vi "SNK3_HF.vi"() -> ()   [LabVIEW 2017]
uses:
  Control_EU/AScan5.ctl
  Control_EU/AScanXY.ctl
  <vilib>/Utility/error.llb/DialogType.ctl
  Control_EU/DataCluster.ctl
  Control_EU/UNDT_ClusterPackRevers (Type).ctl
  E:/_git/LV_Unicorn/Control/unicorn_Param.ctl
  E:/_git/LV_Unicorn/Control/unicorn_conn.ctl
  E:/_git/LV_Unicorn/Control/unicorn_JSON.ctl
  E:/_git/LV_Unicorn/Control/unicorn_ParamInt.ctl
  E:/_git/LV_Unicorn/Control/unicorn_Telemetry.ctl
  E:/_git/LV_Unicorn/Control/unicorn_Table.ctl
  E:/_git/LV_Unicorn/Control/unicorn_ParamFloat.ctl
  Control_EU/UNDT_Graph (Type).ctl
  Control_EU/MeasControl2.ctl
  Control_EU/FilterCor (Type).ctl
  <vilib>/Utility/miscctls.llb/LVPositionTypeDef.ctl
  <vilib>/Utility/miscctls.llb/LVBoundsTypeDef.ctl
  <vilib>/Utility/miscctls.llb/LVRowAndColumnTypeDef.ctl
  E:/_git/LV_Unicorn/LV_Unicorn.lvlib
panel:
  out "Table":string[][](table)
  out "Overload":bool[](array[boolean])
  in  "ScaleAbciss":enum16{"Время", "Растояние"}(ring) caption="Ось X"
  in  "AutoScaleTime":bool=TRUE caption="Автомасштаб оси X"
  out "AScanXY":T1 caption="XY Graph - Light"
  out "AScan 2":T2=[{"f0"=0.0, "df"=1.999999987845058e-08, "magnitude"=[-8.362428618581513, -16.48524282862701, -13.270215291464396, -1.44247262127071, -0.14146356256599724, -51.99620101896437, -99.78053816073843, -95.12827294380126, -90.88869610452232, -90.57171306559249, -87.25341160556846, -85.8105891846696, -82.76337415652955, -80.86227527247217, -78.40234828439452, -76.19434956898783, -74.01576834598359, -71.78529755390673, -69.68513234090051, -67.52084604331412, -65.28443000252219, -63.28035098812552, -61.47587187035788, -55.13083503627922, -33.66107495355482, -4.448097020118439, 6.700743833810975, -2.283159610513394, -7.84886632585858, 20.366429733203404, 85.31206280454444, 128.55518730024505, 126.6691916223117, 121.44842700443678, 120.34183392161685, 117.1312140668606, 115.09733972218146, 112.07993143953263, 109.58979749310856, 106.99556091118939, 104.39191050125919, 101.93090119993394, 99.39922086918887, 96.97715585938386, 94.53860842694485, 92.13340433368103, 89.79334219186057, 87.4974982431977, 84.36064872487259, 79.96205068879135, 75.24407280826563, 69.6830936007591, 63.012279743985346, 56.68454128407484, 50.848901457596185, 45.15521557730699, 39.80757945206551, 34.87529947330404, 30.326640668357868, 25.873379055661644, 21.437604126664155, 17.226033165145054, 13.29233985936753, 9.51676315482473, 5.868301535314458, 2.6152379190580177, -0.17432084983738605, -2.9230732928817815, -5.72915589706281, -8.184331474023566, -10.351473082454504, -12.583499883397053, -14.78807691482325, -16.80357569484977, -18.681385196647625, -20.315395063160395, -21.635529485686448, -23.060485075707675, -24.67995225859704, -25.990605155052435, -26.962380226163987, -27.8979823545651, -28.73810296071838, -29.462829936045352, -30.316506058786985, -31.231589134722654, -31.90290135924215, -32.28940013073094, -32.56549527286779, -32.84419147253834, -33.10821799085829, -33.304481879338255, -33.46348407210644, -33.725072745996385, -33.968450151919114, -34.08677302658134, -34.095260888540906, -33.808795901495614, -33.460191943170685, -33.34710648415603, -33.31294418132484, -33.164550879301714, -32.76087185762208, -32.24668349645117, -31.870751672834558, -31.59434042822022, -31.322524907283878, -30.987392928483132, -30.54575777807395, -29.960390802933034, -29.194569385082104, -28.35521615897005, -27.62954955178202, -27.16065053686043, -26.837023014710212, -26.337914212675514, -25.71672342288184, -25.366631450281602, -25.0282208409094, -24.10622696739074, -22.93802219334293, -22.196530061297835, -21.860867523784236, -21.48748057143621, -20.868178290548485, -20.258140316942672, -19.741215960041927, -19.043028419689563, -18.327886007838515, -17.88242873042077, -17.410982641516057, -16.751452435353258, -16.108829161595168, -15.466698716435872, -14.79714242030252, -14.15875938689237, -13.51766704991087, -13.037019622874197, -12.883695422881942, -12.688494826915928, -12.003125979495529, -11.041384732025477, -10.084146598250413, -9.094988080956, -8.456447500145373, -8.350068617135094, -8.081518682681917, -7.434963428810079, -6.886095277938921, -6.459481766096815, -6.006742309917172, -5.620911678318862, -5.31553427736344, -4.833348073185789, -4.023214092920625, -3.34493790122724, -3.164730433913519, -2.9873376703399117, -2.3525611732443394, -1.6414614161376448, -1.1393857023135752, -0.7026244223184221, -0.32843603777837416, 0.05392266421858949, 0.5455805395231437, 1.1545903160676971, 1.781017592099488, 2.1783846355274363, 2.3977169397439866, 2.665823543012266, 2.9966959607709214, 3.26432535821732, 3.308674526046161, 3.253305179315248, 3.4221076308822376, 3.869108561619214, 4.335963537628231, 4.5814517046546825, 4.784279759130186, 5.183043868629284, 5.453526093130677, 5.427387813380847, 5.645768572191628, 6.244742510133619, 6.7991138215475075, 7.095702891390829, 7.047903714554195, 7.022261210930083, 7.424905424799363, 7.751004705825835, 7.762319244342507, 7.964564695372246, 8.341866396149271, 8.5654588424768, 8.684667654972145, 8.910024715720283, 9.320113816427693, 9.681328111244511, 9.82042605812967, 9.932776687086516, 10.142521316622151, 10.358957614276733, 10.506859328193968, 10.57077349352403, 10.546141368829922, 10.328487343140296, 10.07575920412637, 10.415274780592881, 11.094160586595535, 11.1505633923789, 10.86742877213328, 10.912559327658528, 11.057356953535418, 11.039702429150566, 10.996767826725772, 11.0376960190315, 11.103126869322296, 11.209970057860119, 11.313258819693147, 11.284415966702, 11.287074491221574, 11.317094694615662, 11.153033313477863, 11.164239905021532, 11.507872766702349, 11.54247437227059, 11.245325654941553, 11.284050122036206, 11.60608735389178, 11.684968277664666, 11.552378091289938, 11.30140977616611, 10.82661768874459, 10.552244657690608, 10.730994969471794, 10.877123869724528, 10.799195529112694, 10.689736112373794, 10.550420705492797, 10.323919095222664, 10.143144721401768, 10.238665189584935, 10.300660044676988, 9.877206661005403, 9.430313941227723, 9.375324885704686, 9.274215891535277, 8.97357832792477, 8.962562153335966, 9.31708468024408, 9.395592837025106, 8.951893496609046, 8.490135195852417, 8.349086505424566, 8.490678117530479, 8.621734183776425, 8.474382694063024, 8.254557446893159, 8.08427593174929, 8.008460564436973, 8.166791542098508, 8.139075587574553, 7.846901022328893, 7.817067734629745, 7.839851256288966, 7.585179076138957, 7.335045937828909, 7.162006690912676, 6.940819550198285, 6.836077513955388, 6.936004569442957, 7.062421923523289, 7.029144812631785, 6.8410717702354304, 6.693133085989757, 6.576838506898639, 6.415406266518403, 6.460329048099084, 6.8260616523512, 7.063685025475934, 6.830997901977753, 6.540760553090877, 6.413424153006417, 5.958987769712621, 5.3708356607021415, 5.388070204628093, 5.699517827597447, 5.705195043963613, 5.641944201379374, 5.799467017764982, 5.970988142689748, 5.807005608165127, 5.3246424658118485, 4.860039317596602, 4.624090649915161, 4.646748362163635, 4.749191009974311, 4.680270924636716, 4.500713930749043, 4.367592408763812, 4.225989613421916, 4.151125465745281, 4.213723680311887, 4.159140027255489, 4.002432062387015, 3.952611752314624, 3.957092286027546, 3.8829357749400515, 3.6539695825686067, 3.4836802273675858, 3.423265760191498, 3.2487988787561335, 3.1556659578109247, 3.1891273339861073, 3.007045679469229, 2.6904212670106062, 2.479388271780408, 2.341186118315818, 2.287069402584166, 2.304384948052757, 2.119308207078575, 1.6629850131757848, 1.4292599067393894, 1.5348852188617457, 1.4873002503245516, 1.3294569906902325, 1.3013776101597614, 1.2726427204106585, 1.1502594846460852, 0.7491829966038495, 0.24296145992775564, 0.21561241826202604, 0.41891116519582283, 0.27361930057122663, 0.05490456389088649, 0.06342031008716731, 0.023829591709727538, -0.12211693620702135, -0.10022365821896528, 0.13808831118331, 0.2572844946789701, -0.038020760019207955, -0.451183307570318, -0.46499836947805306, -0.17207548691658303, -0.11017842560977442, -0.3275198146511684, -0.46812528558439226, -0.4643833141108189, -0.35511715348184225, -0.2316420424176613, -0.24180173921013193, -0.28982339790672995, -0.40532542428081797, -0.5930137058367109, -0.66422549393792, -0.7359407593976357, -0.7426463673255057, -0.5872296669112984, -0.5528867670263935, -0.6206878161829081, -0.6536080379892155, -0.5933601194583389, -0.4043312653657267, -0.34505391499988036, -0.4973056554072173, -0.6806381473443253, -0.8142567518480064, -0.7602558335283902, -0.6034238278398334, -0.6499078635251863, -0.8511098952358225, -1.0372637329319332, -1.0373002243404699, -0.8003105749385213, -0.7355750021488348, -0.9524111472992445, -1.150236596544346, -1.209007262785235, -1.1337058391754908, -1.1860405047445965, -1.4007784850109601, -1.536762599852409, -1.6860273416677956, -1.6924470009635115, -1.4112204348384694, -1.3699058167276235, -1.7008180109278328, -1.9213176048579044, -2.110995081726287, -2.3202647740099565, -2.0249377193167675, -1.5526853836036025, -1.5086623250890625, -1.6033312274894342, -1.8652128730554978, -2.4902599231427303, -2.9286209145266184, -2.8737155718090435, -2.6342273377531455, -2.4779406172337985, -2.535840186173118, -2.6692602695266032, -2.589781662843052, -2.4953836821823643, -2.700424055835356, -2.9828725086108534, -3.0823670179938745, -3.0936821349923775, -3.045846607479234, -2.89969529082191, -2.8673928842927126, -2.8816708087679217, -2.654989520570325, -2.4880829681678733, -2.6582434162510253, -2.8447974560167495, -2.835933851381469, -2.792141705112954, -2.844217979802579, -2.906390653235121, -2.86229991317623, -2.7575688328979595, -2.604821473637003, -2.4683593096679033, -2.5354120137767495, -2.6219441167590958, -2.52585252828203, -2.3582229980534066, -2.0089848048764907, -1.589152812267912, -1.6895458889016481, -2.3193483221029965, -2.7390600744138283, -2.5632325668843805, -2.3299278921913356, -2.3886126672950923, -2.3424710799840796, -2.3113094003665537, -2.544097375845922, -2.6177735194071374, -2.4038119720510167, -2.104478329481708, -1.8769032436987345, -1.8297884165408504, -1.8397176026994657, -1.9241985213398038, -2.172246434820863, -2.3580485310660606, -2.350211338635063, -2.2969404170673897, -2.266134637073719, -2.1596259798795927, -2.0569351767576336, -2.1042590716192535, -2.1498693061028007, -2.259218623822335, -2.5957630417007067, -2.8766772717946196, -2.7582052913397774, -2.249975786520963, -1.9910433550871858, -2.2452515904476513, -2.4381017241790914, -2.4313391339662758, -2.226923331641842, -1.9012009420130198, -2.024960099043483, -2.4015471209291945, -2.4217247349968716, -2.398582307210802, -2.5954482817147664, -2.637866804554733, -2.4530357145601442, -2.264939520810856, -2.2922411154767133, -2.6196098565765737, -2.901625679773872, -2.878426945936468, -2.608991094906088, -2.2387857641482753, -2.09453085314685, -2.204732517612733, -2.2719190011368156, -2.3166224061620517, -2.286914558026254, -2.1429486168223733, -2.3244217551271618, -2.688567341423635, -2.5972807503556226, -2.216139264306605, -1.9378262417934877, -1.7862010187935766, -1.8305964693306578, -1.9965156460901028, -2.086063208620317, -1.9612220244869718, -1.6455034137032385, -1.5811718615387917, -1.781927054860887, -1.7300633286956213, -1.5254276131966549, -1.4552768078465874, -1.4523745520051534, -1.4914536016906368, -1.5893559168812885, -1.6015688051501797, -1.3944289829226477, -1.2666103232660362, -1.388013237006021, -1.4446035143943163, -1.4962791866852285, -1.6908152736442617, -1.7476937379832407, -1.5876830010743106, -1.2777607982993686, -1.017954355658162, -1.1298205385137408, -1.2730121585939287, -1.0632148179361138, -0.8644639282300659, -1.0099510796040931, -1.3206230134837824, -1.5056142446026115, -1.4862541127040458, -1.3769159774615218, -1.2309918205446593, -1.0234725791449364, -0.9411732883463628, -0.9697684889927132, -0.9517257621215549, -1.0898865632028674, -1.3386563353294605, -1.4914969798998072, -1.5830446476098814, -1.5645732343650707, -1.4580894296914266, -1.3227021722798327, -1.2047299034683192, -1.3215155550166173, -1.482586656757917, -1.359866040902034, -1.1772395757790264, -0.9929342830718042, -0.8774222730518204, -1.1099924327160124, -1.3080030773072622, -1.2084609742055363, -1.2499391622181975, -1.5056830886296666, -1.4185389284449457, -0.9615123969335855, -0.7803563936448654, -0.9576656839298039, -1.2740004999209305, -1.5303181849230896, -1.4469397956454486, -1.2210108533554376, -1.0927434475643167, -1.0887609884819085, -1.1768500340380115, -1.1383812615431452, -0.899624876448911, -0.7467888409761372, -0.8332742820899739, -0.9191905856778249, -0.8735255850086787, -0.620948668965184, -0.20360162817735272, -0.004829021887644558, -0.06126518615371879, -0.1206794575970207, -0.13042972371681572, -0.14361233031024767, -0.23623177455158384, -0.3409376971964093, -0.37580386508943775, -0.3756449052634707, -0.30167336121257904, -0.15735143907022575, -0.18575377039746854, -0.5125215808075154, -0.6710384180156552, -0.40567774298176573, -0.2658003113576797, -0.3670234725342425, -0.3873427200990136, -0.5013808185888138, -0.6775818427701097, -0.7093324148102056, -0.6240102187909997, -0.31594965771523675, -0.056491991648499607, -0.3432900902159872, -0.7960975868587639, -0.6535675952762858, -0.22854146809868325, -0.29192425843518777, -0.5485119771361724, -0.538319443776345, -0.567697080604944, -0.648059770870077, -0.4951732810517342, -0.2539965079262174, -0.1450610284459799, -0.3003100969881416, -0.7128360258332123, -1.079760020695403, -1.0787566074927781, -0.6326880874656808, -0.10784068463988206, 0.0343957311192753, -0.06698642450328407, -0.13309667361363609, -0.3163761163689287, -0.5315324135831361, -0.3813514187557985, -0.054354728121325024, -0.01385841181718206, -0.16997792231552467, -0.3121017327842992, -0.3990411551312718, -0.36364339922238287, -0.3396735727582154, -0.3071585842604918, -0.010359696911223182, 0.14511950447445088, -0.2589224126552381, -0.5762151230680956, -0.43965938793621717, -0.24733515444995646, -0.19387261615293028, -0.3351491608715378, -0.34532398299666056, -0.027889339253533763, 0.12939961103563746, 0.056654333865026274, 0.1230607529222425, 0.18840971818906382, 0.023524623384787446, 0.007162268968954777, 0.23430478795387444, 0.2837222544059159, 0.17897281281159394, 0.031042575950152695, -0.32807431300739154, -0.7136821519388832, -0.6748008976255733, -0.3134642003245176, -0.005201762167928337, 0.28332615312939424, 0.4825814929413923, 0.4382697634825945, 0.3363950751918878, 0.33043354091955734, 0.4245915317824256, 0.49330159180635746, 0.4035130214653009, 0.24375024460977102, 0.11354505150364957, 0.02126287245380354, -0.053544948000080694, -0.13859926601122652, -0.0724822990500229, 0.20118154548850953, 0.2683717810496091, -0.02587055520410786, -0.3496768753386732, -0.41745076228284006, -0.16421334153824318, 0.12033453428193752, 0.25209620468524463, 0.28430791817811496, 0.18264540514900318, 0.049018916363763765, 0.0016300540045790513, 0.0181018425878392, -0.012450352299282486, -0.26050342961477213, -0.6106594874185305, -0.5902151022163196, -0.16157144082393415, 0.1913050218443857, 0.3467194083880827, 0.3594821624047597, 0.25514771482377796, 0.14863756867879374, 0.02526945654861379, -0.030411099402272157, -0.057532872068520646, -0.1678352196447861, 0.0050842552622896164, 0.4679356219693602, 0.4775913842308057, 0.03565776707866064, -0.02192071464214962, 0.3637345593877086, 0.5089700224787066, 0.21595635766497878, -0.08851796028834258, -0.11535308413340317, 0.07008582549362075, 0.3172098958150116, 0.42725851306396123, 0.19434939967916165, -0.17960096836732475, -0.22300681125435062, 0.03684553140349678, 0.23990696494710662, 0.23882353609518603, 0.2197403890365326, 0.3719346251314626, 0.5769936938241691, 0.5824062303123618, 0.3189435134705114, 0.12519266613720959, 0.16463577053156797, 0.19030497718591022, 0.13549962363308055, 0.13201797751310806, 0.23932364475072632, 0.35005152851859833, 0.3373705359796446, 0.20432943219903166, 0.052721705922394335, 0.10298776022501954, 0.3701207427268116, 0.5430249736029396, 0.5009148342087713, 0.2978760718557538, 0.09219321070600017, 0.13393330859835828, 0.33953567960239184, 0.43052035242115494, 0.38148098994517454, 0.415351558669272, 0.4582932174478742, 0.3124023389633237, 0.17299399106730107, -0.07635904591123222, -0.5307978843140688, -0.5929384987070989, -0.20434243019323617, 0.030884435369358698, -0.011348368912109663, 0.0029669081454244406, 0.14538493119147233, 0.21417009991179725, 0.31184163814498334, 0.371777860209761, 0.1056468743233836, -0.14466540253590665, -0.18406641780580912, -0.32792074087453216, -0.26237246641650813, 0.2894105244412515, 0.6608584286579742, 0.5052543644725347, 0.1611669455267588, -0.12816430138968826, -0.19007337823893522, 0.07215810742349049, 0.5163022496016083, 0.7510023125434486, 0.5472167454923351, 0.32134272812413656, 0.31761231132520606, 0.18537161733263474, 0.03675229199535579, 0.2337274456237992, 0.4585991394025086, 0.3415603897793176, 0.09129735788513926, 0.0756513488759083, 0.21255672357818867, 0.09540049811892004, -3.0665706674426474e-05, 0.2852105377101566, 0.3755848838875977, 0.2018957983494829, 0.1774616682042165, 0.06773902100451323, 0.04379244419664019, 0.3463110501602955, 0.3871378118556663, 0.1833799034141066, 0.2670117046574205, 0.3980808418215247, 0.4290106422002964, 0.458031160928158, 0.27521104721830625, 0.12677865244972963, 0.35520975234021535, 0.5952039721412348, 0.42272504463551286, 0.16031661647281226, 0.21580758179447912, 0.2812243238033716, 0.21902584997582153, 0.3035538101453312, 0.3863830045150394, 0.2917921304942297, 0.28192564587595825, 0.3600489951124928, 0.29434435160408157, 0.1764079844710409, 0.15126766455074403, 0.1763195440069012, 0.04668268981527035, -0.3192578279350755, -0.46618615472317515, -0.14601272298170898, 0.11839185082453696, 0.046519034135144466, -0.042003371722159955, 0.1733477203089251, 0.34455614839816917, -0.07812140797659595, -0.4820299265186918, -0.365581182070855, -0.3375999362822881, -0.5159617905794676, -0.4801205776030315, -0.0732860204226995, 0.4390020279794271, 0.5500131027357611, 0.3648195836488526, 0.20158268236087906, 0.052373137554127425, 0.04563646472297478, 0.05242342103815645, -0.05843066410290021, 0.12945128198407474, 0.5201484582841545, 0.526558984370638, 0.2815502865862527, 0.1492985192964511, 0.10739855659323894, 0.09861915156182022, -0.04135048827669152, -0.35717774361660304, -0.49062788692197046, -0.3209427930853508, 0.016743293250272018, 0.45027484979311794, 0.6216169483678868, 0.4066347156396546, 0.27828313162228824, 0.4707579866840206, 0.6751239786804035, 0.5663001391731655, 0.2615591431004418, 0.14383809871912945, 0.27329166712002007, 0.3410492437734547, 0.3084481169778428, 0.4179537195461194, 0.6732638998383322, 0.8377463664749598, 0.6077008571803617, 0.12627074749883604, -0.030575282680729288, 0.019599161533733422, -0.10365977653168557, -0.12553792707120692, -0.0769794053737769, -0.1637377197200749, -0.09915977471496262, 0.045841608370267295, 0.14535723523528077, 0.3531225340724973, 0.2927312182763444, -0.08970625436268165, -0.15144323159029227, 0.038091603654322626, 0.18762153296160022, 0.3619296478664751, 0.2715231920734027, 0.07013930077545183, 0.20351536174541707, 0.2577293424268987, -0.02410580504505333, -0.2208582024454131, -0.24358480952264472, -0.29277281265297006, -0.316985698973383, -0.20252234111882217, -0.029825552761167273, 0.07774714092482782, 0.11932168624412043, 0.11986880273639144, 0.024756918557329755, -0.20753617553964432, -0.31491271309062085, -0.12032840126028077, 0.01836648590835921, -0.017545829771620447, 0.04954906309080798, 0.1353245450206373, 0.015480990582943832, -0.14787166808844177, -0.057943116083833957, 0.23473363006445425, 0.4173171072892501, 0.512254784727304, 0.6156594232339785, 0.4157091926279577, -0.059021886098150844, -0.2608760366894103, -0.1091841671644147, -0.053648216270971716, -0.11989447865158809, -0.04507068097427691, -0.06597328023218552, -0.2045302059898404, 0.06697666428232196, 0.4984994216806058, 0.384164441988446, 0.016536383149343692, -0.04917977024359743, 0.08319316914810315, 0.08657038669196027, -0.13275948959216066, -0.2077937299213204, 0.007552074793011343, 0.10345140142192122, 0.01329369268262326, 0.08062963424987402, 0.2863543156377659, 0.20276990257247007, -0.13826596361974453, -0.2547753602261764, -0.08288696976654819, 0.08417466470160662, 0.06835279501615332, 0.044575476585407614, 0.033416567190897695, -0.1368734589356677, -0.21416558183864254, -0.1492720501744884, -0.06898489334548685, -0.07289999506372169, -0.26528800995998836, -0.21049792023552527, 0.013814347194966103, -0.09401329989805163, -0.262602759939341, -0.2616421759547052, -0.10424188169645277, 0.10439958779164726, 0.175354545824689, 0.2173334881438791, 0.19286862516662495, 0.1412484277265662, 0.12012481576584833, -0.15301161441982458, -0.4815057561094136, -0.45341131556318715, -0.1445173348590174, 0.1663094149535027, 0.2099185189720174, -0.07742022745577515, -0.41168006577396454, -0.45924723795656064, -0.2756570382527457, -0.17081435490473496, -0.1693257181831882, -0.0786346890587879, 0.15919665769553148, 0.3773983729545307, 0.3759213188999979, 0.09973732479323871, -0.17066898838561428, 0.027740917095059103, 0.34729937252632226, 0.18999857876508486, -0.10778459345812053, -0.23149832753205146, -0.17943298052233558, 0.10809672363149048, 0.37739306215007673, 0.5303181336562943, 0.5814618677817407, 0.3888715199087187, 0.10232232585565271, -0.13786434062996022, -0.24750633688256585, -0.1203930974364198, -0.04723627025555288, -0.1252965541626736, -0.046062891273265905, 0.15716680469029143, 0.216832061463208, -0.08796584481672198, -0.4652283810208928, -0.2605998533882712, 0.10981870056053822, -0.003628019655366188, -0.08618401606685211, 0.09732282934305658]}, ...(72 in all)]
  in  "FreqFind":dbl=-1.0 caption="Частота, МГц" min=-1.0 max=10000000.0 format="%_3f"
  out "UNDT_meas":string[][](table)=[["Частота, Гц", "1", "-", "-"], ["СКЗ, В", "1", "-", "-"], ["Амплитуда, В", "1", "-", "-"], ["Амплитуда, дБмкВ", "1", "-", "-"], ["Датчик пути 1, мм", "1", "-", "-"], ["Датчик пути 2, мм", "1", "-", "-"], ["Время, сек", "1", "-", "-"]]
  in  "Tab":enum32{"Параметры общие", "Отладка", "K"}(tab)=enum."K"
  in  "Автозапрос телеметри":bool
  in  "Тип детектора":enum16{"Оконный детектор", "Гильберт"}(ring)=enum."Гильберт"
  in  "FiltrCor":bool caption="Поправка на АЧХ фильтра"
  in  "speed":dbl=1500.0 caption="скорость звука, м/с"
  in  "DelaiProtector":dbl[](array[numeric])=[0.0, 0.0, 0.0, 0.0, 0.0, 0.0, 0.0, 0.0, 0.0, 0.0, 0.0, 0.0, 0.0, 0.0, 0.0, 0.0, 0.0, 0.0, 0.0, 0.0, 0.0, 0.0, 0.0, 0.0, 0.0, 0.0, 0.0, 0.0, 0.0, 0.0, 0.0, 0.0, 0.0, 0.0, 0.0, 0.0, 0.0, 0.0, 0.0, 0.0, 0.0, 0.0, 0.0, 0.0, 0.0, 0.0, 0.0, 0.0, 0.0, 0.0, 0.0, 0.0, 0.0, 0.0, 0.0, 0.0, 0.0, 0.0, 0.0, 0.0, 0.0, 0.0, 0.0, 0.0] caption="Задержка в проетекторе, мкс"
  out "HPF_Bode":cluster{"Frq":dbl[], "Kt":dbl[]}[](graph)=[{"Frq"=[100000.0, 200000.0, 300000.0, 400000.0, 500000.0, 600000.0, 700000.0, 800000.0, 900000.0, 1000000.0, 1100000.0, 1200000.0, 1300000.0, 1400000.0, 1500000.0, 2000000.0, 3000000.0, 4000000.0, 5000000.0, 6000000.0, 7000000.0, 8000000.0, 9000000.0, 10000000.0, 11000000.0, 12000000.0, 13000000.0, 14000000.0, 15000000.0], "Kt"=[0.37286, 0.79297, 0.90962, 0.95419, 0.97594, 0.98749, 0.98845, 0.99808, 1.00096, 1.00096, 1.00192, 1.00192, 1.00289, 1.00289, 1.00192, 1.0, 0.98653, 0.96728, 0.94447, 0.91646, 0.8898, 0.85438, 0.80953, 0.76035, 0.69865, 0.62859, 0.54832, 0.46631, 0.38142]}, {"Frq"=[100000.0, 200000.0, 300000.0, 400000.0, 500000.0, 600000.0, 700000.0, 800000.0, 900000.0, 1000000.0, 1100000.0, 1200000.0, 1300000.0, 1400000.0, 1500000.0, 2000000.0, 3000000.0, 4000000.0, 5000000.0, 6000000.0, 7000000.0, 8000000.0, 9000000.0, 10000000.0, 11000000.0, 12000000.0, 13000000.0, 14000000.0, 15000000.0], "Kt"=[0.3742, 0.79565, 0.91266, 0.95739, 0.97874, 0.99034, 0.9971, 1.00097, 1.00386, 1.0029, 1.00483, 1.00483, 1.00483, 1.00483, 1.00386, 1.0, 0.98068, 0.94986, 0.90947, 0.85923, 0.79836, 0.72744, 0.6486, 0.56483, 0.47855, 0.39459, 0.31478, 0.24271, 0.18]}, {"Frq"=[100000.0, 200000.0, 300000.0, 400000.0, 500000.0, 600000.0, 700000.0, 800000.0, 900000.0, 1000000.0, 1100000.0, 1200000.0, 1300000.0, 1400000.0, 1500000.0, 2000000.0, 3000000.0, 4000000.0, 5000000.0, 6000000.0, 7000000.0, 8000000.0, 9000000.0, 10000000.0, 11000000.0, 12000000.0, 13000000.0, 14000000.0, 15000000.0], "Kt"=[0.37978, 0.80756, 0.9262, 0.97125, 0.99215, 1.00393, 1.01079, 1.01374, 1.01178, 1.01472, 1.01472, 1.01472, 1.01374, 1.01178, 1.01079, 1.0, 0.96222, 0.90903, 0.84171, 0.76408, 0.67763, 0.58508, 0.49117, 0.3999, 0.31452, 0.23886, 0.17399, 0.12139, 0.08052]}, {"Frq"=[100000.0, 200000.0, 300000.0, 400000.0, 500000.0, 600000.0, 700000.0, 800000.0, 900000.0, 1000000.0, 1100000.0, 1200000.0, 1300000.0, 1400000.0, 1500000.0, 2000000.0, 3000000.0, 4000000.0, 5000000.0, 6000000.0, 7000000.0, 8000000.0, 9000000.0, 10000000.0, 11000000.0, 12000000.0, 13000000.0, 14000000.0, 15000000.0], "Kt"=[1.0, 1.0, 1.0, 1.0, 1.0, 1.0, 1.0, 1.0, 1.0, 1.0, 1.0, 1.0, 1.0, 1.0, 1.0, 1.0, 1.0, 1.0, 1.0, 1.0, 1.0, 1.0, 1.0, 1.0, 1.0, 1.0, 1.0, 1.0, 1.0]}, {"Frq"=[], "Kt"=[]}]
  in  "Захват потока":bool
  out "IndCntr":u32
  in  "BasePathData":path=path "D:/YandexDisk/!Work/_labview/SNK3/data"
  in  "ZeroDimensionDetect":i32=10
  out "MD5_filter_ini":string="528970cebd473443910cf3af22e246ff"
  in  "UNDT_HF_Filter":u16=7 caption="ФВЧ аппаратный" max=10 step=1
  in  "I_AMP1_PE2":i32
  in  "I_AMP1_PE1":i32
  out "ScaleADC":bool=TRUE
  in  "StartLen":T3={"start samples/time"=0.0, "duration"=7e-05, "EnableSubset"=FALSE}
  out "LPF_Bode":cluster{"Frq":dbl[], "Kt":dbl[]}[](graph)=[{"Frq"=[100000.0, 200000.0, 300000.0, 400000.0, 500000.0, 600000.0, 700000.0, 800000.0, 900000.0, 1000000.0, 1100000.0, 1200000.0, 1300000.0, 1400000.0, 1500000.0, 2000000.0, 3000000.0, 4000000.0, 5000000.0, 6000000.0, 7000000.0, 8000000.0, 9000000.0, 10000000.0, 11000000.0, 12000000.0, 13000000.0, 14000000.0, 15000000.0], "Kt"=[0.37335, 0.7928, 0.90924, 0.95331, 0.97471, 0.98638, 0.99416, 0.99805, 1.00097, 1.0, 1.00195, 1.00195, 1.00195, 1.00195, 1.00195, 1.0, 0.98735, 0.96848, 0.94484, 0.91946, 0.89125, 0.86021, 0.82772, 0.79426, 0.75934, 0.72539, 0.69066, 0.65661, 0.62296]}, {"Frq"=[100000.0, 200000.0, 300000.0, 400000.0, 500000.0, 600000.0, 700000.0, 800000.0, 900000.0, 1000000.0, 1100000.0, 1200000.0, 1300000.0, 1400000.0, 1500000.0, 2000000.0, 3000000.0, 4000000.0, 5000000.0, 6000000.0, 7000000.0, 8000000.0, 9000000.0, 10000000.0, 11000000.0, 12000000.0, 13000000.0, 14000000.0, 15000000.0], "Kt"=[0.37335, 0.7928, 0.90924, 0.95331, 0.97471, 0.98638, 0.99416, 0.99805, 1.00097, 1.0, 1.00195, 1.00195, 1.00195, 1.00195, 1.00195, 1.0, 0.98735, 0.96848, 0.94484, 0.91946, 0.89125, 0.86021, 0.82772, 0.79426, 0.75934, 0.72539, 0.69066, 0.65661, 0.62296]}, {"Frq"=[100000.0, 200000.0, 300000.0, 400000.0, 500000.0, 600000.0, 700000.0, 800000.0, 900000.0, 1000000.0, 1100000.0, 1200000.0, 1300000.0, 1400000.0, 1500000.0, 2000000.0, 3000000.0, 4000000.0, 5000000.0, 6000000.0, 7000000.0, 8000000.0, 9000000.0, 10000000.0, 11000000.0, 12000000.0, 13000000.0, 14000000.0, 15000000.0], "Kt"=[0.37335, 0.7928, 0.90924, 0.95331, 0.97471, 0.98638, 0.99416, 0.99805, 1.00097, 1.0, 1.00195, 1.00195, 1.00195, 1.00195, 1.00195, 1.0, 0.98735, 0.96848, 0.94484, 0.91946, 0.89125, 0.86021, 0.82772, 0.79426, 0.75934, 0.72539, 0.69066, 0.65661, 0.62296]}, {"Frq"=[100000.0, 200000.0, 300000.0, 400000.0, 500000.0, 600000.0, 700000.0, 800000.0, 900000.0, 1000000.0, 1100000.0, 1200000.0, 1300000.0, 1400000.0, 1500000.0, 2000000.0, 3000000.0, 4000000.0, 5000000.0, 6000000.0, 7000000.0, 8000000.0, 9000000.0, 10000000.0, 11000000.0, 12000000.0, 13000000.0, 14000000.0, 15000000.0], "Kt"=[0.37335, 0.7928, 0.90924, 0.95331, 0.97471, 0.98638, 0.99416, 0.99805, 1.00097, 1.0, 1.00195, 1.00195, 1.00195, 1.00195, 1.00195, 1.0, 0.98735, 0.96848, 0.94484, 0.91946, 0.89125, 0.86021, 0.82772, 0.79426, 0.75934, 0.72539, 0.69066, 0.65661, 0.62296]}, {"Frq"=[100000.0, 200000.0, 300000.0, 400000.0, 500000.0, 600000.0, 700000.0, 800000.0, 900000.0, 1000000.0, 1100000.0, 1200000.0, 1300000.0, 1400000.0, 1500000.0, 2000000.0, 3000000.0, 4000000.0, 5000000.0, 6000000.0, 7000000.0, 8000000.0, 9000000.0, 10000000.0, 11000000.0, 12000000.0, 13000000.0, 14000000.0, 15000000.0], "Kt"=[0.20101, 0.60917, 0.79214, 0.87772, 0.9244, 0.95111, 0.96794, 0.97883, 0.98639, 0.98962, 0.99325, 0.99567, 0.99728, 0.99849, 0.99919, 1.0, 0.98871, 0.97006, 0.94536, 0.91804, 0.8877, 0.85474, 0.82046, 0.78558, 0.7497, 0.71522, 0.68054, 0.64677, 0.61381]}, {"Frq"=[100000.0, 200000.0, 300000.0, 400000.0, 500000.0, 600000.0, 700000.0, 800000.0, 900000.0, 1000000.0, 1100000.0, 1200000.0, 1300000.0, 1400000.0, 1500000.0, 2000000.0, 3000000.0, 4000000.0, 5000000.0, 6000000.0, 7000000.0, 8000000.0, 9000000.0, 10000000.0, 11000000.0, 12000000.0, 13000000.0, 14000000.0, 15000000.0], "Kt"=[0.20101, 0.60917, 0.79214, 0.87772, 0.9244, 0.95111, 0.96794, 0.97883, 0.98639, 0.98962, 0.99325, 0.99567, 0.99728, 0.99849, 0.99919, 1.0, 0.98871, 0.97006, 0.94536, 0.91804, 0.8877, 0.85474, 0.82046, 0.78558, 0.7497, 0.71522, 0.68054, 0.64677, 0.61381]}, {"Frq"=[100000.0, 200000.0, 300000.0, 400000.0, 500000.0, 600000.0, 700000.0, 800000.0, 900000.0, 1000000.0, 1100000.0, 1200000.0, 1300000.0, 1400000.0, 1500000.0, 2000000.0, 3000000.0, 4000000.0, 5000000.0, 6000000.0, 7000000.0, 8000000.0, 9000000.0, 10000000.0, 11000000.0, 12000000.0, 13000000.0, 14000000.0, 15000000.0], "Kt"=[0.20101, 0.60917, 0.79214, 0.87772, 0.9244, 0.95111, 0.96794, 0.97883, 0.98639, 0.98962, 0.99325, 0.99567, 0.99728, 0.99849, 0.99919, 1.0, 0.98871, 0.97006, 0.94536, 0.91804, 0.8877, 0.85474, 0.82046, 0.78558, 0.7497, 0.71522, 0.68054, 0.64677, 0.61381]}, {"Frq"=[100000.0, 200000.0, 300000.0, 400000.0, 500000.0, 600000.0, 700000.0, 800000.0, 900000.0, 1000000.0, 1100000.0, 1200000.0, 1300000.0, 1400000.0, 1500000.0, 2000000.0, 3000000.0, 4000000.0, 5000000.0, 6000000.0, 7000000.0, 8000000.0, 9000000.0, 10000000.0, 11000000.0, 12000000.0, 13000000.0, 14000000.0, 15000000.0], "Kt"=[0.20101, 0.60917, 0.79214, 0.87772, 0.9244, 0.95111, 0.96794, 0.97883, 0.98639, 0.98962, 0.99325, 0.99567, 0.99728, 0.99849, 0.99919, 1.0, 0.98871, 0.97006, 0.94536, 0.91804, 0.8877, 0.85474, 0.82046, 0.78558, 0.7497, 0.71522, 0.68054, 0.64677, 0.61381]}]
  in  "ScaleOrdinate":T4(ring)=enum."Вольты" caption="Ось ординат"
  out "Log":string="[8:41:50] Запуск ПО СНК3. Версия 2.0.30032026. Цифровой идентификатор (MD5):  .\r\n"
  in  "SaveParam":bool
  in  "GainCompens":bool
  out "Ошибка":bool
  in  "UDPDataInd0":bool
  in  "save_osc":bool[](array[boolean])
  in  "index_osc":i32=32
  in  "Refresh":bool
  in  "RingMenu":u16(ring) items=["Основные параметры", "Данные", "Параметры фильтра", "Прочее"]
  in  "TabRight":enum32{"Page 1", "Page 4", "Page 3", "Page 2"}(tab)
  in  "TxPulseCh0":u8=1 caption="№ ПЭП подкл. к ГИВ" min=1 max=16 step=1
  in  "TxPulseCh1":u8=1 caption="Кол-во имп. ГИ" min=1 max=16 step=1
  in  "HPF_Filter_Prog":T5(ring)=enum."Выкл." caption="ФВЧ"
  in  "TxDelay1":dbl caption="t задержки имп., мкс" min=0.0 max=30.0 step=0.05 format="%.2g"
  in  "TxCh0":u8=1 caption="№ ПЭП подкл. к ГИВ" min=1 max=8 step=1
  in  "WPulse0":dbl=0.4000000059604645 caption="t импульса, мкс" min=0.05 max=1.0 step=0.01 format="%.2g"
  in  "Tx0":bool=TRUE caption="Разрешить работу генератора"
  in  "TxDelay0":dbl caption="t задержки имп. , мкс" min=0.0 max=30.0 step=0.05 format="%.2g"
  in  "Tick":i32=1 caption="№ такта" min=1 max=32 step=1
  in  "TxCh1":u8=16 caption="№ ПЭП подкл. к ГИ" min=9 max=16 step=1
  in  "Tx1":bool=TRUE caption="Разрешить работу генератора"
  in  "PWhite1":dbl=0.4000000059604645 caption="t импульса, мкс" min=0.05 max=1.0 step=0.01 format="%_2g"
  in  "RxCh0":u8=1 caption="№ ПЭП подкл. к приемнику" min=1 max=8 step=1
  in  "RxDelay0":dbl caption="t задержки разв. , мкс" min=0.0 max=200.0 step=1.0
  in  "RxCh1":u8=9 caption="№ ПЭП подкл. к приемнику" min=9 max=16 step=1
  in  "RxDelay1":dbl caption="t задержки разв. , мкс" min=0.0 max=200.0 step=1.0
  in  "Rx0":bool=TRUE caption="Разрешить работу приемника"
  in  "Rx1":bool=TRUE caption="Разрешить работу приемника"
  in  "RxWhite0":dbl=20.0 caption="t разв. , мкс" min=1.0 max=80.0
  in  "RxWhite1":dbl=20.0 caption="t разв. , мкс" min=1.0 max=80.0
  in  "Gain1":dbl caption="Усиление, дБ" min=0.0 max=80.0 step=1.0
  in  "Gain0":dbl caption="Усиление, дБ" min=0.0 max=80.0 step=1.0
  in  "UNDT_Mean":i32=4 caption="Усреднение по времени" min=0 max=28 step=4
  in  "UNDT_NTick":i32=1 caption="Количество тактов" min=1 max=32 step=1
  in  "UNDT_Freq":i32=100 caption="Частота следования тактов, Гц" min=20 max=1000 step=1
  in  "UNDT_GIV2":T6(ring)=enum."60" caption="Амплитуда ГИВ2 (ПЭП 9...16), В"
  in  "UNDT_GIV1":T6(ring)=enum."60" caption="Амплитуда ГИВ1 (ПЭП 1...8), В"
  in  "Type_signal":T7(ring)
  in  "LPF_Filter":enum16{"14 МГц", "10 МГц", "7.5 МГц"}(ring) caption="ФНЧ"
  in  "Видеофильтр":bool=TRUE
  in  "TrigLevel":dbl=0.1 caption="Уровень триггера" min=-1.0 max=10000000.0 format="%_3f"
  in  "IIR filter":T8={"Topology"=enum."Butterworth", "Type"=enum."Bandpass", "Order"=4, "Lower Fc"=300000.0, "Upper Fc"=15000000.0, "PB Ripple"=3.0, "SB Attenuation"=60.0} {"PB Ripple" format="%0.2f"; "SB Attenuation" format="%0.2f"; "Lower Fc" format="%0.2p"; "Upper Fc" format="%0.2p"}
  in  "IndEnqu":enum16{"NoEnqu", "LossyEnqu", "Enqu"}(ring)=enum."LossyEnqu"
  in  "Interpolation factor (n)":i32=1
  in  "Ind":bool=TRUE
  in  "max queue size":i32=4
  out "UpTime":sgl
  in  "Connect":bool
  in  "Save":bool
  in  "Pause":bool
  in  "UNDT_Start":bool
  # "График 1"
  # "График 2"
  # "График 3"
  # "График 4"
  # "График 5"
  # "График 6"
  # "График 7"
  # "График 8"
  # "ПЭП 1...8"
  # "ПЭП 9...16"
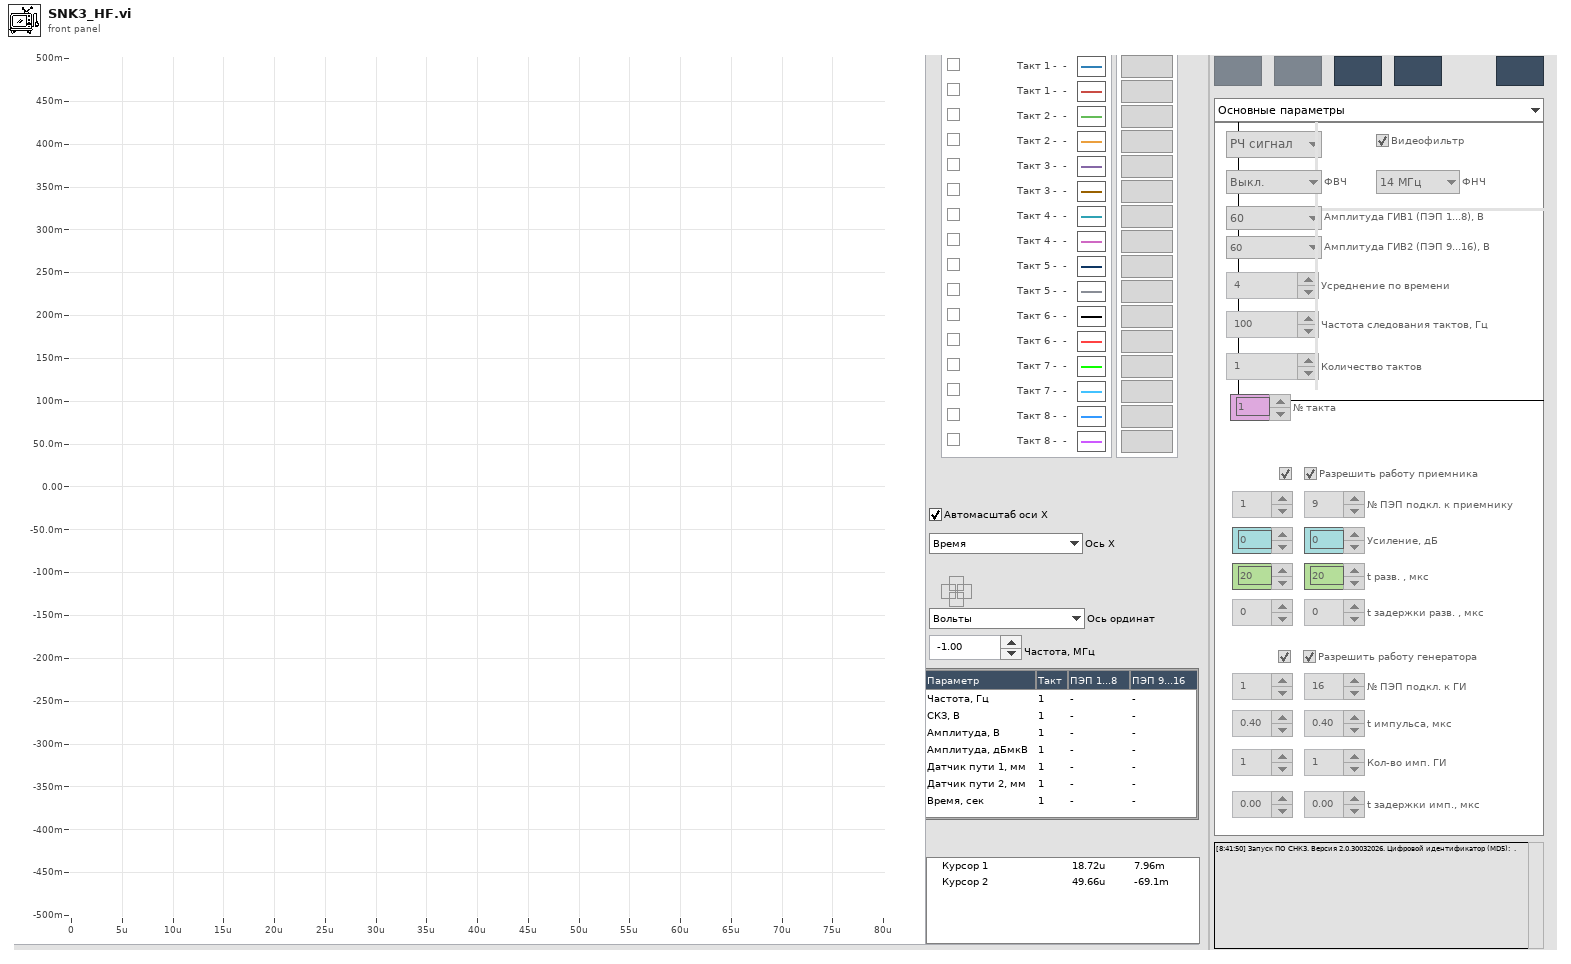
[diagram p1: front panel]
types:
  T1 = typedef "AScanXY.ctl" = cluster{dbl[], dbl[]}[]
  T2 = typedef "AScan5.ctl" = cluster{"f0":dbl, "df":dbl, "magnitude":dbl[]}[]
  T3 = cluster{"start samples/time":dbl, "duration":dbl, "EnableSubset":bool}
  T4 = enum16{"Отсчеты АЦП (±32767)", "Проценты", "Вольты", "дБмкВ (отн. 1 мкВ)", "Отсчеты АЦП (±1)"}
  T5 = enum16{"0.4 МГц", "0.8 МГц", "1.5 МГц", "2.0 МГц", "Выкл."}
  T6 = enum16{"20", "40", "60", "80", "100", "120", "140", "160", "180", "200"}
  T7 = enum16{"РЧ сигнал", "Детект. полное", "Положит.", "Отрицат."}
  T8 = cluster{"Topology":enum16{"Off", "Butterworth", "Chebyshev", "Inverse Chebyshev", "Elliptic", "Bessel"}, "Type":enum16{"Lowpass", "Highpass", "Bandpass", "Bandstop"}, "Order":i32, "Lower Fc":dbl, "Upper Fc":dbl, "PB Ripple":dbl, "SB Attenuation":dbl}
  T9 = typedef "LV_Unicorn.lvlib/unicorn_Param.ctl" = cluster{"conParam":T10, "Param":T11}
  T10 = typedef "LV_Unicorn.lvlib/unicorn_conn.ctl" = cluster{"ReadIntParam":bool, "ReadDescrParam":bool, "ReadFloatParam":bool, "debug":bool, "ReadJSON":bool, "IP_address":string, "N_attempts":i32, "type_con":enum16{"Serial", "TCP"}, "MB_address":i32, "VISA":refnum<visa-resource-name>, "connection ID":refnum<k5>, "nameDevices":string, "timeout":i32, "port":u16, "type_version":string, "baud_rate":u32, "VersionControl":bool, "TCP_conn":bool, "WindowSize":i32}
  T11 = typedef "LV_Unicorn.lvlib/unicorn_JSON.ctl" = cluster{"NumParam":cluster{"NTelem":i32, "NInt":i32, "NFloat":i32, "NTable":i32}, "ParamInt":T12, "Telemetry":T13, "Table":T14, "ParamFloat":T15}
  T12 = typedef "LV_Unicorn.lvlib/unicorn_ParamInt.ctl" = cluster{"ID":string, "Num":i32, "Name":string, "Type":string, "Enum":string, "Desc":string, "Unit":string, "Access":string, "FormatStr":string, "Min":i32, "Max":i32}[]
  T13 = typedef "LV_Unicorn.lvlib/unicorn_Telemetry.ctl" = cluster{"ID":string, "Num":i32, "Name":string, "Desc":string, "Unit":string, "FormatStr":string, "Min":i32, "Max":i32}[]
  T14 = typedef "LV_Unicorn.lvlib/unicorn_Table.ctl" = cluster{"Num":i32, "Access":string, "ColumnCount":i32, "NeedParamPrepare":bool, "Columns":cluster{"Column":i32, "Desc":string, "Name":string}[], "DataType":string, "FormatStr":string, "ID":string, "Name":string, "RowCount":i32, "Rows":cluster{"Desc":string, "ID":string, "Max":i32, "Min":i32, "Name":string, "Row":i32, "Unit":string}[], "Type":string}[]
  T15 = typedef "LV_Unicorn.lvlib/unicorn_ParamFloat.ctl" = cluster{"ID":string, "Num":i32, "Name":string, "Type":string, "Enum":string, "Desc":string, "Unit":string, "Access":string, "FormatStr":string, "Min":sgl, "Max":sgl}[]
  T16 = typedef "DataCluster.ctl" = cluster{"UNDT_Cluster":T17, "UNDT_Cluster_Data":dbl[]}
  T17 = typedef "UNDT_ClusterPackRevers (Type).ctl" = cluster{"PacketCounter":u32, "Gain Coeff":sgl, "SamplingInterval":sgl, "Lose Packet":u32, "EncodersParam2":u64, "EncodersParam1":u64, "Reserve 1":u8, "Mux TX/RX":u8, "ScanDelay":u16, "CRC 8":u8, "ScanDuration":u16, "N chanel":u8, "GlobalTime2":u32, "GlobalTime1":u32, "N tick":u8, "Ncycle":u16, "FrameFormatVersion":u8, "MagicWord":u32, "Overload":bool}
  T18 = typedef "DialogType.ctl" = u16
  T19 = enum8{"Enabled", "Disabled", "Disabled and Grayed Out"}
  T20 = typedef "LVRowAndColumnTypeDef.ctl" = cluster{"Row":i32, "Column":i32}
  T21 = cluster{"Версия:":string, "Наименование ПО:":string, "Год выпуска:":string, "Производитель:":string, "MD5":string, "Наименование ПО полное:":string, "Build":string}
  T22 = typedef "ConfigINI.ctl" = cluster{"IP_PC":string, "IP_SNK3":string, "UDP_port_0":u32, "UDP_port_1":u32, "Serial_Code":string, "ADCToVoltage0":dbl, "DelayChN":dbl[], "GainCorrection":dbl[][], "CorCh":dbl[], "PulseCor":dbl[][], "ADCToVoltage1":dbl}
  T23 = typedef "OptionPACK5.ctl" = cluster{"MagicWordStr":string, "Header size":u32, "Проверка CRC8":bool, "Проверка конца пакета":bool, "GainCompens":bool, "Неотбрасывать BadEnd пакеты":bool, "Неотбрасывать BadCRC пакеты":bool, "Привести к 1":bool, "GainCoef":bool, "K_scale":dbl, "ScaleOrdinate":enum16{"Отсчеты АЦП (±32767)", "Проценты", "Вольты", "дБмкВ (отн. 1 мкВ)", "Отсчеты АЦП (±1)"}}
  T24 = enum16{"Отсчеты АЦП ", "Отсчеты АЦП приведенные к ±1", "Вольты", "дБмкВ (отн. 1 мкВ)"}
  T25 = typedef "LVPositionTypeDef.ctl" = cluster{"Left":i32, "Top":i32}
  T26 = typedef "LVBoundsTypeDef.ctl" = cluster{"Width":u32, "Height":u32}
  T27 = typedef "LVRangeTypeDef.ctl" = cluster{"Minimum":dbl, "Maximum":dbl, "Increment":dbl, "Minor Increment":dbl, "Start":dbl}
  T28 = typedef "LVRectTypeDef.ctl" = cluster{"Left":i16, "Top":i16, "Right":i16, "Bottom":i16}
  T29 = typedef "FilterCor (Type).ctl" = cluster{"HPFFilterNum":enum16{"HPF_OFF", "1", "2", "3", "4", "5", "6", "7", "8", "9", "10"}, "LPFBode":cluster{"Frq":dbl[], "Kt":dbl[]}[], "HPFBode":cluster{"Frq":dbl[], "Kt":dbl[]}[], "EnableFilterСorrect":bool, "LPF_Filter":enum16{"14 МГц", "10 МГц", "7.5 МГц", "Выкл."}}
  T30 = typedef "MeasControl2.ctl" = cluster{"approx freq":dbl, "search (+/- % of Fsampl.)":dbl, "start, duration":cluster{"start samples/time":dbl, "duration":dbl, "EnableSubset":bool}, "averaging type":enum16{"Linear", "Exponential"}, "window":enum16{"Rectangular (none)", "Hanning", "Low side lobe"}, "hysteresis":dbl, "level":dbl}
  T31 = typedef "UNDT_Graph (Type).ctl" = cluster{"UNDT_Type_signal":enum16{"РЧ сигнал", "Детект. полное", "Положит.", "Отрицат."}, "ФНЧ":bool, "UNDT_Mean":i32, "IIR filter":cluster{"Topology":enum16{"Off", "Butterworth", "Chebyshev", "Inverse Chebyshev", "Elliptic", "Bessel"}, "Type":enum16{"Lowpass", "Highpass", "Bandpass", "Bandstop"}, "Order":i32, "Lower Fc":dbl, "Upper Fc":dbl, "PB Ripple":dbl, "SB Attenuation":dbl}, "ZeroDimension":i32, "ТипДетектора":enum16{"Оконный детектор", "Гильберт"}, "FilterCor":cluster{"HPFFilterNum":enum16{"HPF_OFF", "1", "2", "3", "4", "5", "6", "7", "8", "9", "10"}, "LPFBode":cluster{"Frq":dbl[], "Kt":dbl[]}[], "HPFBode":cluster{"Frq":dbl[], "Kt":dbl[]}[], "EnableFilterСorrect":bool, "LPF_Filter":enum16{"14 МГц", "10 МГц", "7.5 МГц", "Выкл."}}, "MeasControl":T30}
  T32 = typedef "MeasControl.ctl" = cluster{"FFT amplitude":dbl, "amplitude":dbl, "RMS":dbl, "detected frequency":dbl, "way sensor 1":ext, "way sensor 2":ext, "detected frequency 2":dbl, "time trig":dbl, "time trig 2":dbl, "DC":dbl, "trigger detected?":bool, "FFT amplitude mean":dbl}
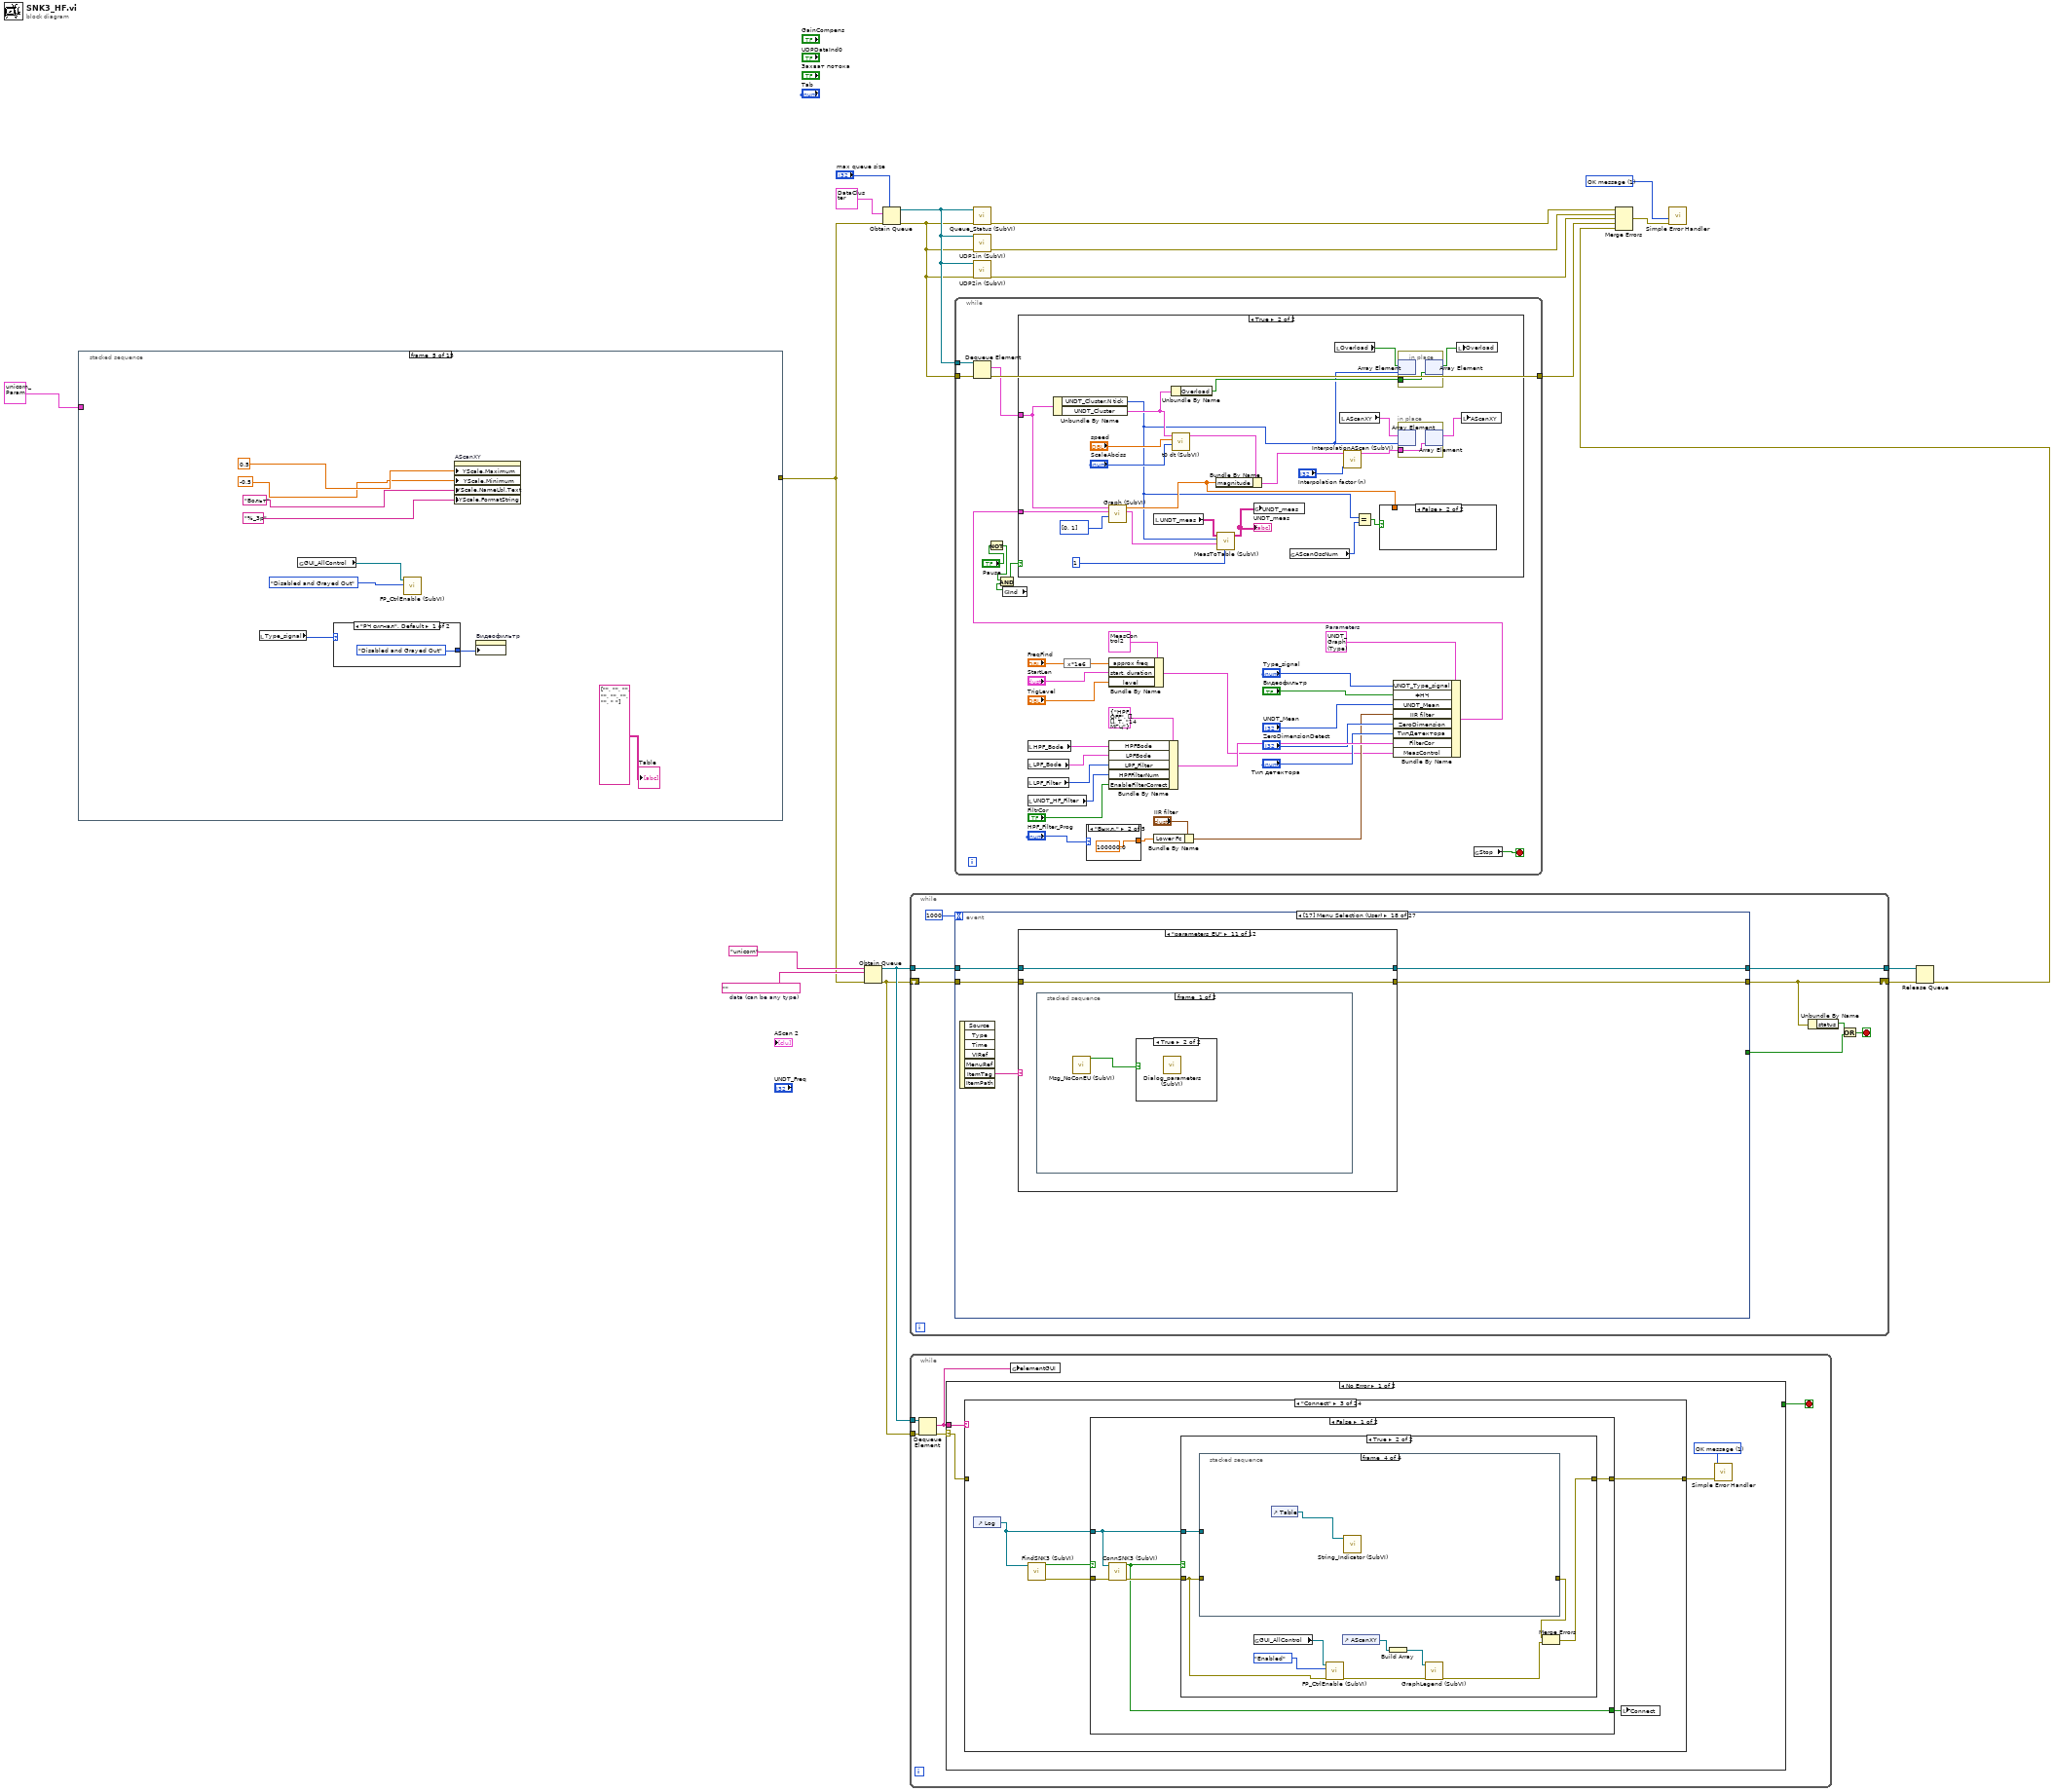
[diagram p0: block diagram]
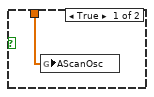
[diagram p3: hidden frame]
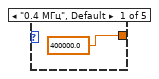
[diagram p4: hidden frame]
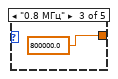
[diagram p5: hidden frame]
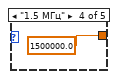
[diagram p6: hidden frame]
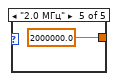
[diagram p7: hidden frame]
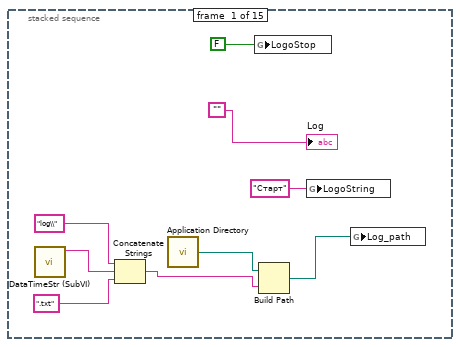
[diagram p8: hidden frame]
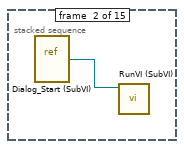
[diagram p9: hidden frame]
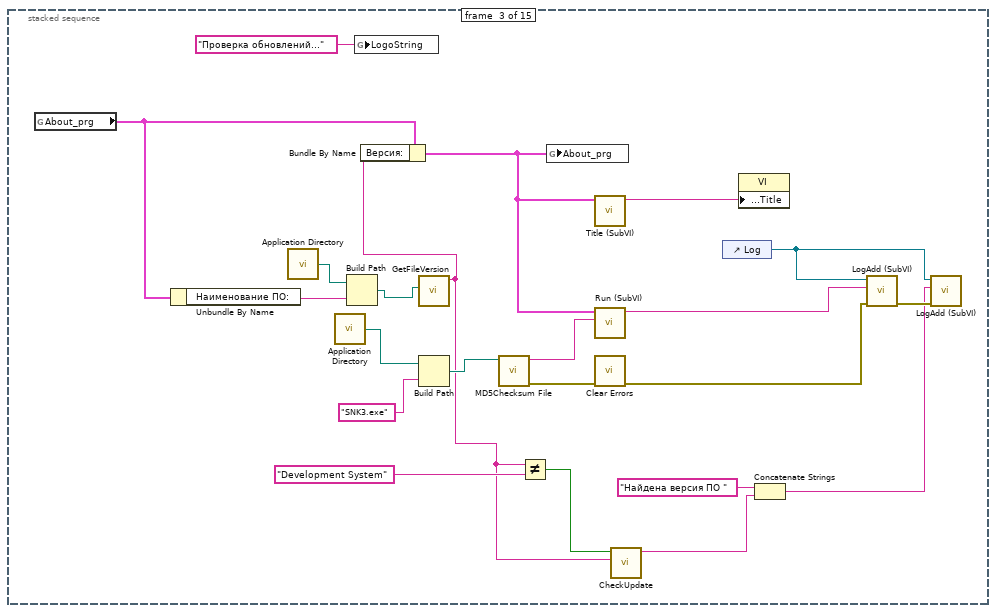
[diagram p10: hidden frame]
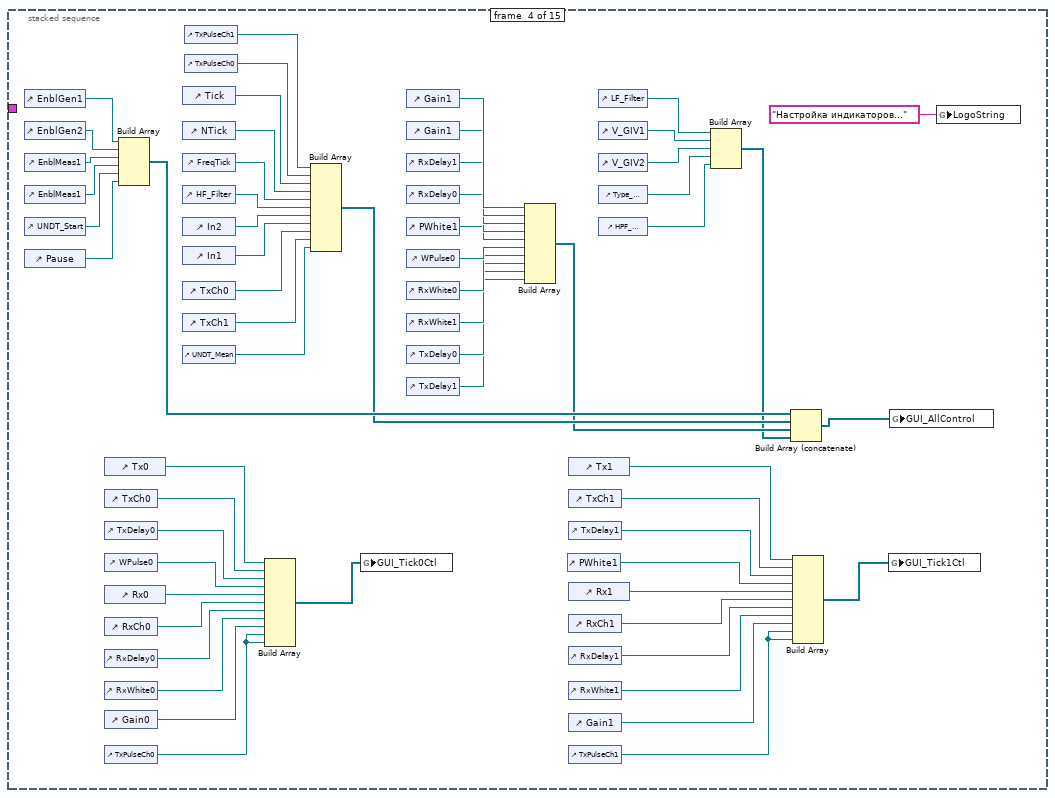
[diagram p11: hidden frame]
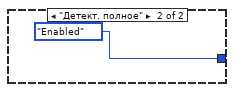
[diagram p12: hidden frame]
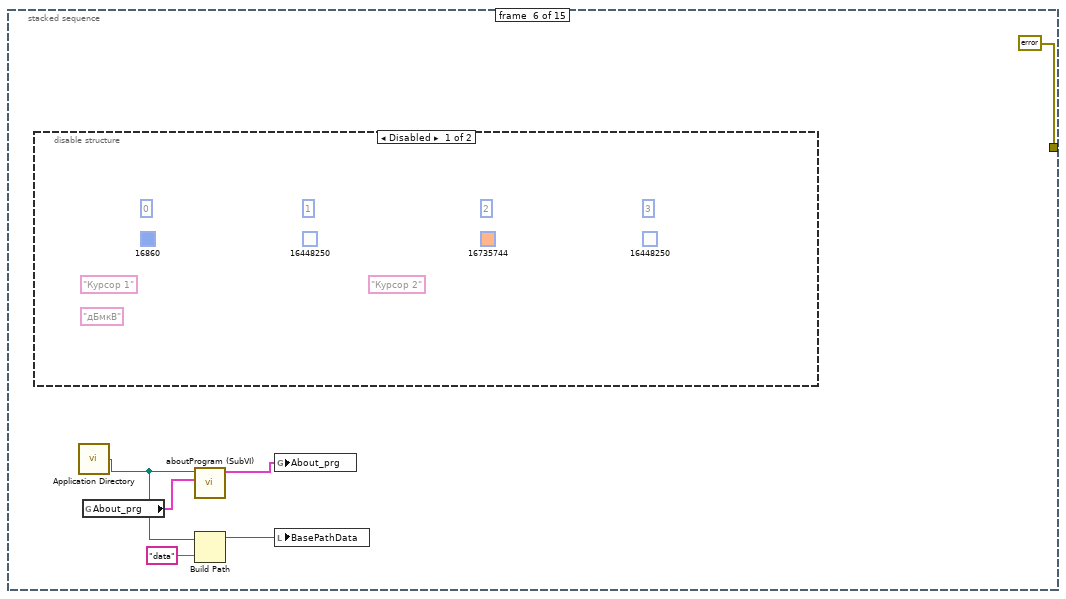
[diagram p13: hidden frame]
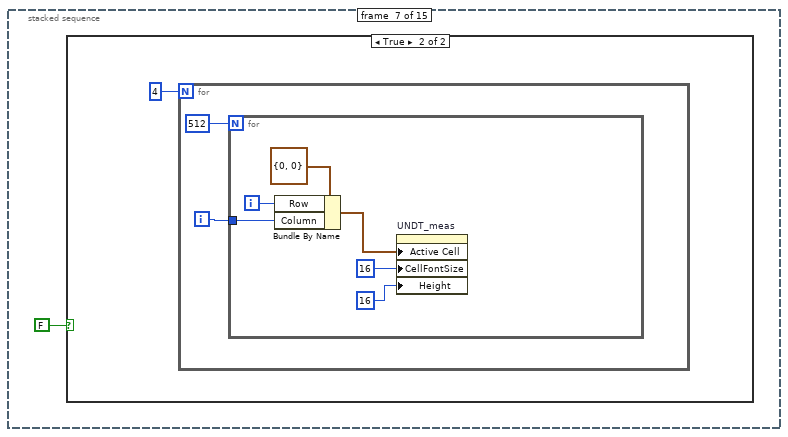
[diagram p15: hidden frame]
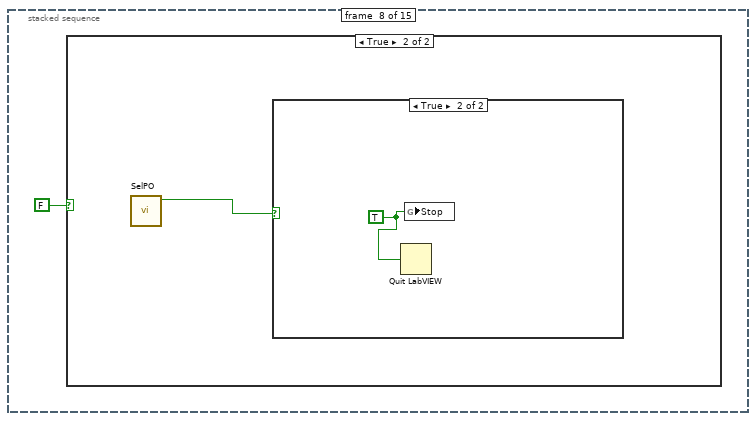
[diagram p17: hidden frame]
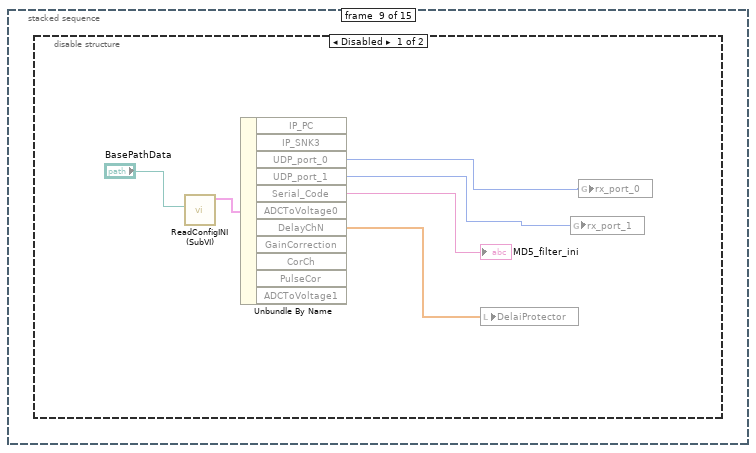
[diagram p20: hidden frame]
diagram:
  w18 = ""  # data (can be any type)
  w19 = T18 1 items=["no dialog", "OK message", "continue or stop message", "OK message + warnings", "continue/stop + warnings"] ("type of dialog (OK msg:1)")
  n1 = stacked-sequence {
    tunnel: [_ _ _ _ _ errorcluster {"status"=FALSE, "code"=0, "source"=""} ("error in (no error)") _ _ _ _ _ _ _ _ _] -> w3
    tunnel: T9 {"conParam"={"ReadIntParam"=TRUE, "ReadDescrParam"=FALSE, "ReadFloatParam"=TRUE, "debug"=FALSE, "ReadJSON"=TRUE, "IP_address"="192.168.1.216", "N_attempts"=5, "type_con"=enum."TCP", "MB_address"=1, "VISA"="COM1", "connection ID"=refnum, "nameDevices"="", "timeout"=2000, "port"=2000, "type_version"="0F0C0005", "baud_rate"=115200, "VersionControl"=TRUE, "TCP_conn"=FALSE, "WindowSize"=700}, "Param"={"NumParam"={"NTelem"=201, "NInt"=16, "NFloat"=10, "NTable"=2}, "ParamInt"=[], "Telemetry"=[], "Table"=[], "ParamFloat"=[]}} ("paramUnicorn") -> [_ _ _ _ _ _ _ _ _ _ w174 _ _ _ _]
    frame #0 {
      n2 = call "DataTimeStr (SubVI).vi"() -> ("DataTimeStr"=w23:string)  [unwired: 11 in]
      n3 = Concatenate Strings("log\\" ("name or relative path"), w23, ".txt" ("name or relative path")) -> (w22:string)
      n4 = call <vilib>:"Application Directory.vi"() -> ("Application Directory"=w24:path)
      n5 = global write "Global_SNK3_HF.vi" "LogoStop"(FALSE ("StopStartLogo")) -> ()
      n6 = Build Path(base path=w24, name or relative path=w22) -> (appended path=w25:path)
      n7 = global write "Global_SNK3_HF.vi" "LogoString"("Старт" ("LogoString")) -> ()
      n8 = global write "Global_SNK3_HF.vi" "Log_path"(w25) -> ()
      "Log" <- ""
    }
    frame #1 {
      n9 = vi-ref "Dialog_Start (SubVI).vi"() -> (w29:refnum<vi>)
      n10 = call "RunVI (SubVI).vi"("VI in"=w29) -> ()  [unwired: 11 in]
    }
    frame #2 {
      n11 = global read "Global_SNK3_HF.vi" "About_prg"() -> (w41:T21)
      n12 = Unbundle By Name(w41) -> ("Наименование ПО:"=w43:string)
      n13 = call <vilib>:"Application Directory.vi"() -> ("Application Directory"=w42:path)
      n14 = call <vilib>:"Application Directory.vi"() -> ("Application Directory"=w49:path)
      n15 = Build Path(base path=w42, name or relative path=w43) -> (appended path=w40:path)
      n16 = global write "Global_SNK3_HF.vi" "LogoString"("Проверка обновлений..." ("LogoString")) -> ()
      n17 = call "GetFileVersion.vi"("path"=w40) -> ("Full version"=w37:string)  [unwired: 10 in]
      n18 = Bundle By Name(cluster=w41, "Версия:"=w37) -> (w44:T21)
      n19 = Build Path(base path=w49, name or relative path="SNK3.exe") -> (appended path=w48:path)
      n20 = call <vilib>:"MD5Checksum File.vi"("Path"=w48) -> ("error out"=w45:errorcluster, "MD5 message-digest"=w47:string)  [unwired: 9 in]
      n21 = Not Equal?(x=w37, y="Development System" ("Full version")) -> (x != y?=w38:bool)
      n22 = global write "Global_SNK3_HF.vi" "About_prg"(w44) -> ()
      n23 = call "Title (SubVI).vi"("About_prg"=w44) -> ("String"=w46:string)  [unwired: 10 in]
      n24 = call "Run (SubVI).vi"("MD5 message-digest"=w47, "About_prg"=w44) -> ("String"=w51:string)  [unwired: 9 in]
      n25 = call <vilib>:"Clear Errors.vi"("error in (no error)"=w45) -> ("error out"=w30:errorcluster)  [unwired: 5 in, 1 out]
      n26 = call "CheckUpdate.vi"("Установленная версия ПО"=w37, "GitHub"=w38) -> ("Последняя версия ПО"=w32:string)  [unwired: 9 in]
      n27 = control-ref of="Log"() -> (w34:refnum<vi>)
      n28 = property class="VI"("Front Panel.Title"=w46) -> ()  [unwired: 2 in, 2 out]
      n29 = Concatenate Strings("Найдена версия ПО " ("string"), w32) -> (w31:string)
      n30 = call "LogAdd (SubVI).vi"("error in"=w30, "string"=w51, "Log"=w34) -> ("error out"=w35:errorcluster)  [unwired: 8 in]
      n31 = call "LogAdd (SubVI).vi"("error in"=w35, "string"=w31, "Log"=w34) -> ()  [unwired: 8 in, 1 out]
    }
    frame #3 {
      n32 = control-ref of="EnblGen1"() -> (w111:refnum<vi>)
      n33 = control-ref of="EnblGen2"() -> (w110:refnum<vi>)
      n34 = control-ref of="EnblMeas1"() -> (w109:refnum<vi>)
      n35 = control-ref of="EnblMeas1"() -> (w108:refnum<vi>)
      n36 = control-ref of="UNDT_Start"() -> (w78:refnum<vi>)
      n37 = control-ref of="Pause"() -> (w77:refnum<vi>)
      n38 = control-ref of="Tx0"() -> (w76:refnum<vi>)
      n39 = control-ref of="TxCh0"() -> (w75:refnum<vi>)
      n40 = control-ref of="TxDelay0"() -> (w74:refnum<vi>)
      n41 = control-ref of="WPulse0"() -> (w73:refnum<vi>)
      n42 = control-ref of="Rx0"() -> (w72:refnum<vi>)
      n43 = control-ref of="RxCh0"() -> (w71:refnum<vi>)
      n44 = control-ref of="RxDelay0"() -> (w70:refnum<vi>)
      n45 = control-ref of="RxWhite0"() -> (w69:refnum<vi>)
      n46 = control-ref of="Gain0"() -> (w68:refnum<vi>)
      n47 = control-ref of="TxPulseCh0"() -> (w54:refnum<vi>)
      n48 = Build Array(w111, w110, w109, w108, w78, w77) -> (w86:refnum<vi>[])
      n49 = control-ref of="Tick"() -> (w107:refnum<vi>)
      n50 = control-ref of="NTick"() -> (w106:refnum<vi>)
      n51 = control-ref of="FreqTick"() -> (w105:refnum<vi>)
      n52 = control-ref of="HF_Filter"() -> (w104:refnum<vi>)
      n53 = control-ref of="In2"() -> (w93:refnum<vi>)
      n54 = control-ref of="In1"() -> (w92:refnum<vi>)
      n55 = control-ref of="TxCh0"() -> (w91:refnum<vi>)
      n56 = control-ref of="TxCh1"() -> (w90:refnum<vi>)
      n57 = control-ref of="UNDT_Mean"() -> (w81:refnum<vi>)
      n58 = control-ref of="TxPulseCh1"() -> (w56:refnum<vi>)
      n59 = control-ref of="TxPulseCh0"() -> (w55:refnum<vi>)
      n60 = Build Array(w76, w75, w74, w73, w72, w71, w70, w69, w68, w54, w54) -> (w67:refnum<vi>[])
      n61 = Build Array(w56, w55, w107, w106, w105, w104, w93, w92, w91, w90, w81) -> (w85:refnum<vi>[])
      n62 = global write "Global_SNK3_HF.vi" "GUI_Tick0Ctl"(w67) -> ()
      n63 = control-ref of="Gain1"() -> (w103:refnum<vi>)
      n64 = control-ref of="Gain1"() -> (w102:refnum<vi>)
      n65 = control-ref of="RxDelay1"() -> (w101:refnum<vi>)
      n66 = control-ref of="RxDelay0"() -> (w100:refnum<vi>)
      n67 = control-ref of="PWhite1"() -> (w99:refnum<vi>)
      n68 = control-ref of="WPulse0"() -> (w98:refnum<vi>)
      n69 = control-ref of="RxWhite0"() -> (w97:refnum<vi>)
      n70 = control-ref of="RxWhite1"() -> (w96:refnum<vi>)
      n71 = control-ref of="TxDelay0"() -> (w95:refnum<vi>)
      n72 = control-ref of="TxDelay1"() -> (w94:refnum<vi>)
      n73 = Build Array(w103, w102, w101, w100, w99, w98, w97, w96, w95, w94) -> (w84:refnum<vi>[])
      n74 = control-ref of="PWhite1"() -> (w62:refnum<vi>)
      n75 = control-ref of="Tx1"() -> (w65:refnum<vi>)
      n76 = control-ref of="TxCh1"() -> (w64:refnum<vi>)
      n77 = control-ref of="TxDelay1"() -> (w63:refnum<vi>)
      n78 = control-ref of="Rx1"() -> (w61:refnum<vi>)
      n79 = control-ref of="RxCh1"() -> (w60:refnum<vi>)
      n80 = control-ref of="RxDelay1"() -> (w59:refnum<vi>)
      n81 = control-ref of="RxWhite1"() -> (w58:refnum<vi>)
      n82 = control-ref of="Gain1"() -> (w57:refnum<vi>)
      n83 = control-ref of="TxPulseCh1"() -> (w53:refnum<vi>)
      n84 = control-ref of="LF_Filter"() -> (w89:refnum<vi>)
      n85 = control-ref of="V_GIV1"() -> (w88:refnum<vi>)
      n86 = control-ref of="V_GIV2"() -> (w87:refnum<vi>)
      n87 = control-ref of="Type_signal"() -> (w80:refnum<vi>)
      n88 = control-ref of="HPF_Filter_Prog"() -> (w79:refnum<vi>)
      n89 = Build Array(w89, w88, w87, w80, w79) -> (w83:refnum<vi>[])
      n90 = Build Array (concatenate)(w86, w85, w84, w83) -> (w82:refnum<vi>[])
      n91 = Build Array(w65, w64, w63, w62, w61, w60, w59, w58, w57, w53, w53) -> (w66:refnum<vi>[])
      n92 = global write "Global_SNK3_HF.vi" "GUI_Tick1Ctl"(w66) -> ()
      n93 = global write "Global_SNK3_HF.vi" "GUI_AllControl"(w82) -> ()
      n94 = global write "Global_SNK3_HF.vi" "LogoString"("Настройка индикаторов..." ("LogoString")) -> ()
    }
    frame #4 {
      n95 = local read "Type_signal"() -> (w117:T7)
      n96 = global read "Global_SNK3_HF.vi" "GUI_AllControl"() -> (w120:refnum<vi>[])
      n97 = case shown="\"РЧ сигнал\", Default" w117 {
        tunnel: [T19."Disabled and Grayed Out" ("Disabled") T19."Enabled" ("Disabled")] -> w118
        frame "РЧ сигнал", Default {
        }
        frame "Детект. полное" {
        }
      }
      n98 = call "FP_CtrlEnable (SubVI).vi"("Disabled"=T19."Disabled and Grayed Out", "Array"=w120) -> ()  [unwired: 9 in, 1 out]
      n99 = property on="AScanXY" class="XYGraph (strict)"("YScale.Maximum"=0.5 ("Y Scale.Range:Maximum"), "YScale.Minimum"=-0.5 ("Y Scale.Range:Minimum"), "YScale.NameLbl.Text"="Вольт" ("Y Scale.Name Label.Text"), "YScale.FormatString"="%_3p" ("Y Scale.Format String")) -> ()  [unwired: 2 in, 2 out]
      n100 = property on="Видеофильтр" class="Bool (strict)"("DisabledEnum"=w118) -> ()  [unwired: 2 in, 2 out]
      "Table" <- string[][] [[""], [""], [""], [""], [""], [""], [""], [" "]] ("Table")
    }
    frame #5 {
      n101 = disable-structure shown="Disabled" {
        frame Disabled {
          w129 = "дБмкВ" ("Cursor.Cursor Name")
          w130 = "Курсор 2" ("Cursor.Cursor Name")
          w131 = "Курсор 1" ("Cursor.Cursor Name")
          w134 = u32 16448250
          w135 = u32 3 ("Active Cursor")
          w133 = u32 16735744
          w132 = u32 2 ("Active Cursor")
          w137 = u32 16448250
          w136 = u32 1 ("Active Cursor")
          w138 = u32 16860
          w139 = u32 0 ("Active Cursor")
        }
        frame Enabled {
        }
      }
      n102 = call <vilib>:"Application Directory.vi"() -> ("Application Directory"=w123:path)
      n103 = global read "Global_SNK3_HF.vi" "About_prg"() -> (w127:T21)
      n104 = call "aboutProgram (SubVI).vi"("About_prg in"=w127, "Application Directory"=w123) -> ("About_prg out"=w126:T21)  [unwired: 9 in]
      n105 = Build Path(base path=w123, name or relative path="data") -> (appended path=w125:path)
      n106 = global write "Global_SNK3_HF.vi" "About_prg"(w126) -> ()
      n107 = local write "BasePathData"(w125) -> ()
    }
    frame #6 {
      n108 = case shown="True" FALSE {
        frame False {
        }
        frame True {
          n109 = for {
            N: 4 -> [_]
            i -> [w142]
            n110 = for {
              N: 512 -> [_]
              tunnel: w142 -> [w146]
              i -> [w147]
              n111 = Bundle By Name(cluster=T20 {"Row"=0, "Column"=0} ("Active Cell:Active Cell"), "Row"=w147, "Column"=w146) -> (w148:T20)
              n112 = property on="UNDT_meas" class="Tbl (strict)"("Active Cell"=w148, "CellFontSize"=u32 16 ("Active Cell:Cell Font:Size"), "Height"=u32 16 ("Active Cell:Cell Size:Height")) -> ()  [unwired: 2 in, 2 out]
            }
          }
        }
      }
    }
    frame #7 {
      n113 = case shown="True" FALSE {
        frame False {
        }
        frame True {
          n114 = call "SelPO.vi"() -> ("AddPOSel"=w151:bool)  [unwired: 10 in, 1 out]
          n115 = case shown="True" w151 {
            frame False {
            }
            frame True {
              w152 = TRUE ("Stop")
              n116 = Quit LabVIEW(quit? (T)=w152) -> ()
              n117 = global write "Global_SNK3_HF.vi" "Stop"(w152) -> ()
            }
          }
        }
      }
    }
    frame #8 {
      n118 = disable-structure shown="Disabled" {
        frame Disabled {
          n119 = call "ReadConfigINI (SubVI).vi"("base path"="BasePathData") -> ("ini cluster"=w157:T22)  [unwired: 10 in]
          n120 = Unbundle By Name(w157) -> ("UDP_port_0"=w153:u32, "UDP_port_1"=w154:u32, "Serial_Code"=→"MD5_filter_ini":string, "DelayChN"=w155:dbl[])  [unwired: 7 out]
          n121 = local write "DelaiProtector"(w155) -> ()
          n122 = global write "Global_SNK3_HF.vi" "rx_port_1"(w154) -> ()
          n123 = global write "Global_SNK3_HF.vi" "rx_port_0"(w153) -> ()
        }
        frame Enabled {
        }
      }
    }
    frame #9 {
      n124 = disable-structure shown="Disabled" {
        frame Disabled {
          n125 = local read "MD5_filter_ini"() -> (w163:string)
          n126 = local read "BasePathData"() -> (w164:path)
          n127 = call "ReadFilterINI (SubVI).vi"("CheckMD5"=FALSE, "base path"=w164, "md5"=w163) -> ("LPF1"=w160:cluster{"Frq":dbl[], "Kt":dbl[]}[], "HPF0"=→"HPF_Bode":cluster{"Frq":dbl[], "Kt":dbl[]}[], "LPF0"=w161:cluster{"Frq":dbl[], "Kt":dbl[]}[])  [unwired: 5 in, 1 out]
          n128 = Insert Into Array(array=w161, new element=w160) -> (→"LPF_Bode":cluster{"Frq":dbl[], "Kt":dbl[]}[])  [unwired: 1 in]
          n129 = for {
            tunnel: w161 -> [w173] mode=indexing
            tunnel: [w170] -> _ mode=indexing
            tunnel: w160 -> [w167] mode=indexing
            tunnel: [w166] -> _ mode=indexing
            n130 = Unbundle By Name(w167) -> ("Frq"=w168:dbl[], "Kt"=w169:dbl[])
            n131 = Unbundle By Name(w173) -> ("Frq"=w172:dbl[], "Kt"=w171:dbl[])
            n132 = Build Array(w172, w171) -> (w170:dbl[][])
            n133 = Build Array(w168, w169) -> (w166:dbl[][])
          }
        }
        frame Enabled {
        }
      }
    }
    frame #10 {
      w180 = T4."Вольты" ("ScaleOrdinate")
      w187 = string[][] [] ("Таблица телеметрии")
      w182 = FALSE ("TCP conn")
      n134 = global read "Global_SNK3_HF.vi" "Spectr_save"() -> (w186:cluster{"f0":dbl, "df":dbl, "magnitude":dbl[]}[])
      n135 = Empty Array?(array=w186) -> (empty?=w188:bool)
      n136 = global write "Global_SNK3_HF.vi" "Stop"(w182) -> ()
      n137 = local write "Автозапрос телеметри"(w182) -> ()
      n138 = local write "Pause"(w182) -> ()
      n139 = local write "UNDT_Start"(w182) -> ()
      n140 = local write "Connect"(w182) -> ()
      n141 = local write "Ошибка"(w182) -> ()
      n142 = case shown="True" w188 {
        frame False {
        }
        frame True {
          n143 = for {
            N: 8 -> [_]
            tunnel: [cluster{"f0":dbl, "df":dbl, "magnitude":dbl[]} {"f0"=0.0, "df"=0.0, "magnitude"=[]} ("magnitude")] -> w192 mode=indexing
          }
          n144 = global write "Global_SNK3_HF.vi" "Spectr_save"(w192) -> ()
        }
      }
      n145 = local write "ScaleOrdinate"(T4."Вольты" ("ScaleOrdinate")) -> ()
      n146 = global read "Global_SNK3_HF.vi" "OptPACKPL1"() -> (w183:T23)
      n147 = global read "Global_SNK3_HF.vi" "OptPACKPL0"() -> (w181:T23)
      n148 = Bundle By Name(cluster=w183, "ScaleOrdinate"=w180) -> (w184:T23)
      n149 = Bundle By Name(cluster=w181, "ScaleOrdinate"=w180) -> (w179:T23)
      n150 = Initialize Array(FALSE, 64 ("dimension size")) -> (→"Overload":bool[])
      n151 = global write "Global_SNK3_HF.vi" "paramUnicorn"(w174) -> ()
      n152 = global write "Global_SNK3_HF.vi" "OptPACKPL1"(w184) -> ()
      n153 = global write "Global_SNK3_HF.vi" "OptPACKPL0"(w179) -> ()
      n154 = global write "Global_SNK3_HF.vi" "IP_PC"("" ("IP_PC")) -> ()
      n155 = global write "Global_SNK3_HF.vi" "TblTelem"(w187) -> ()
      n156 = global write "Global_SNK3_HF.vi" "TblInt"(w187) -> ()
      n157 = global write "Global_SNK3_HF.vi" "AScanOscNum"(u8 255 ("AScanOscNum")) -> ()
      "ScaleADC" <- TRUE ("ScaleADC")
      "IndCntr" <- u32 0 ("UDPLostPack")
    }
    frame #11 {
      n158 = local read "UNDT_NTick"() -> (w197:i32)
      n159 = local read "ScaleOrdinate"() -> (w195:T4)
      n160 = call "TableCollum(SubVI).vi"("ScaleOrdinate 2"=w195, "UNDT_NTick"=w197) -> ("array"=w196:string[][])  [unwired: 9 in]
      n161 = local write "UNDT_meas"(w196) -> ()
    }
    frame #12 {
      n162 = for {
        N: 64 -> [_]
        i -> [w200]
        n163 = Quotient & Remainder(x=w200, y=2) -> (floor(x/y)=w201:i32)  [unwired: 1 out]
        n164 = Increment(x=w201) -> (x+1=w206:i32)
        n165 = Number To Decimal String(number=w206) -> (decimal integer string=w205:string)  [unwired: 1 in]
        n166 = case shown="0, Default" w201 {
          tunnel: [" -   " ("string") " -   " ("string")] -> w202
          frame 0, Default {
          }
          frame 1 {
          }
        }
        n167 = Concatenate Strings("Такт " ("string"), w205, " - " ("string"), w202) -> (w199:string)
        n168 = property on="AScanXY" class="XYGraph (strict)"("Active Plot"=w200, "Plot.Plot Name"=w199) -> ()  [unwired: 2 in, 2 out]
      }
    }
    frame #13 {
      n169 = control-ref of="AScanXY"() -> (w210:refnum<vi>)
      n170 = Initialize Array(cluster{dbl[], dbl[]} {[], []} ("XY Graph"), 72 ("dimension size")) -> (→"AScanXY":cluster{dbl[], dbl[]}[])
      n171 = call "Refresh_AScan (SubVI).vi"("WaveformGraph in"=w210) -> ()  [unwired: 10 in, 1 out]
    }
    frame #14 {
      n172 = global write "Global_SNK3_HF.vi" "LogoString"("Загрузка заверщина" ("LogoString")) -> ()
      n173 = global write "Global_SNK3_HF.vi" "LogoStop"(TRUE ("StopStartLogo")) -> ()
    }
  }
  n174 = Obtain Queue(name (unnamed)="unicorn", element data type=w18, error in (no error)=w3) -> (queue out=w4:refnum<queue>, error out=w2:errorcluster)  [unwired: 2 in, 1 out]
  n175 = Obtain Queue(max queue size (-1, unlimited)="max queue size", element data type=T16 {"UNDT_Cluster"={"PacketCounter"=0, "Gain Coeff"=0.0, "SamplingInterval"=0.0, "Lose Packet"=0, "EncodersParam2"=0, "EncodersParam1"=0, "Reserve 1"=0, "Mux TX/RX"=0, "ScanDelay"=0, "CRC 8"=0, "ScanDuration"=0, "N chanel"=0, "GlobalTime2"=0, "GlobalTime1"=0, "N tick"=0, "Ncycle"=0, "FrameFormatVersion"=0, "MagicWord"=0, "Overload"=FALSE}, "UNDT_Cluster_Data"=[]} ("output cluster 2"), error in (no error)=w3) -> (queue out=w10:refnum<queue>, error out=w7:errorcluster)  [unwired: 2 in, 1 out]
  n176 = while {
    tunnel: w4 -> [w222]
    shift-right: [w218] -> w17
    shift-left: w2 -> [w221]
    tunnel: [w216] -> w5
    stop <- w217 stop-if-true
    n177 = event shown="[17] Menu Selection (User)" {
      selector: _ -> [_ _ _ _ _ _ _ _ _ _ _ _ _ _ _ _ _ _ _ _ _ _ _ _ _ _ _]
      dyn-events: _ -> [_ _ _ _ _ _ _ _ _ _ _ _ _ _ _ _ _ _ _ _ _ _ _ _ _ _ _]
      timeout: 1000 -> [_ _ _ _ _ _ _ _ _ _ _ _ _ _ _ _ _ _ _ _ _ _ _ _ _ _ _]
      tunnel: [w243 _ _ _ _ _ _ _ _ _ _ _ _ _ _ _ _ _ _ _ _ _ _ _ _ _ _] -> w219
      tunnel: w222 -> [w239 _ w267 w295 w300 w312 w324 w338 w351 w386 w427 w454 w466 w529 w571 w580 w619 w622 w686 w705 w717 w722 w734 w775 w802 w829 w845]
      tunnel: w221 -> [w240 _ w266 w294 w299 w311 w323 w337 w350 w385 w419 w453 w471 w527 w572 w579 w618 w621 w684 w703 w716 w721 w731 w776 w801 w823 w844]
      tunnel: [w241 _ w264 w293 w298 w310 w322 w335 w349 w384 w417 w449 w461 w518 w572 w578 w617 w620 w683 w704 w715 w720 w730 w776 w799 w807 w844] -> w218
      tunnel: [w242 _ w267 w287 w297 w309 w321 w336 w348 w383 w423 w450 w460 w517 w571 w575 w619 w623 w679 w705 w713 w718 w734 w775 w798 w829 w845] -> w216
      event Timeout {
        n178 = event-data() -> ()  [unwired: 1 in, 3 out]
        n179 = Get Queue Status(queue=w239, error in (no error)=w240) -> (queue out=w238:refnum<queue>, error out=w237:errorcluster, # elements in queue=w236:i32, elements=w235:string[])  [unwired: 5 out]
        n180 = case shown="0" w236 {
          tunnel: [w245 w249] -> w242
          tunnel: [w244 w248] -> w241
          tunnel: w238 -> [w245 w247]
          tunnel: w237 -> [w244 w246]
          frame 1, Default {
          }
          frame 0 {
            n181 = Enqueue Element(queue=w247, element="Core uptime", error in (no error)=w246) -> (queue out=w251:refnum<queue>, error out=w252:errorcluster)  [unwired: 1 in, 1 out]
            n182 = case shown="True" "Автозапрос телеметри" {
              tunnel: w251 -> [w254 w259]
              tunnel: w252 -> [w255 w258]
              tunnel: [w255 w257] -> w248
              tunnel: [w254 w256] -> w249
              frame False {
              }
              frame True {
                n183 = Enqueue Element(queue=w259, element="Telem", error in (no error)=w258) -> (queue out=w256:refnum<queue>, error out=w257:errorcluster)  [unwired: 1 in, 1 out]
              }
            }
          }
        }
        n184 = global read "Global_SNK3_HF.vi" "UDP0_packet_speed"() -> (w233:dbl)
        n185 = global read "Global_SNK3_HF.vi" "UDP1_packet_speed"() -> (w234:dbl)
        n186 = global write "Global_SNK3_HF.vi" "#el_queue GUI"(w236) -> ()
        n187 = global write "Global_SNK3_HF.vi" "elementsGUI"(w235) -> ()
        n188 = Add(x=w233, y=w234) -> (x+y=w232:dbl)
        n189 = Number To Fractional String(number=w232, precision (6)=i16 1) -> (F-format string=w230:string)  [unwired: 2 in]
        n190 = Concatenate Strings(w230, " Мбит/с" ("string")) -> (w225:string)
        n191 = local read "Table"() -> (w228:string[][])
        n192 = Replace Array Subset(array=w228, new element=w225, index (row)=1 ("disabled index (row)"), index (col)=0 ("disabled index (col)")) -> (w224:string[][])
        n193 = local write "Table"(w224) -> ()
        n194 = global read "Global_SNK3_HF.vi" "Stop"() -> (w243:bool)
      }
      event "IndEnqu": Value Change {
        n195 = event-data() -> ()  [unwired: 1 in, 6 out]
        n196 = global write "Global_SNK3_HF.vi" "IndEnqu"("IndEnqu") -> ()
      }
      event "Type_signal": Value Change {
        n197 = event-data() -> ("NewVal"=w273:T7)  [unwired: 1 in, 5 out]
        n198 = local read "ScaleOrdinate"() -> (w276:T4)
        n199 = Equal?(x=T7."РЧ сигнал" ("NewVal"), y=w273) -> (x = y?=w271:bool)
        n200 = Equal?(x=w276, y=T24."дБмкВ (отн. 1 мкВ)" ("ScaleOrdinate")) -> (x = y?=w272:bool)
        n201 = And(x=w272, y=w271) -> (x .and. y?=w270:bool)
        n202 = case shown="False" w270 {
          tunnel: [w283 w284] -> w269
          frame False {
            n203 = local read "ScaleOrdinate"() -> (w283:T4)
          }
          frame True {
            w284 = T4."Вольты" ("ScaleOrdinate")
            n204 = local write "ScaleOrdinate"(w284) -> ()
          }
        }
        n205 = case shown="True" FALSE {
          tunnel: [0.0 w282] -> w278
          frame False {
          }
          frame True {
            n206 = local read "Gain1"() -> (w281:dbl)
            n207 = local read "Gain0"() -> (w280:dbl)
            n208 = Max & Min(x=w281, y=w280) -> (max(x,y)=w282:dbl)  [unwired: 1 out]
          }
        }
        n209 = case shown="\"РЧ сигнал\", Default" w273 {
          tunnel: [T19."Disabled and Grayed Out" ("Disabled") T19."Enabled" ("Disabled")] -> w277
          frame "РЧ сигнал", Default {
          }
          frame "Детект. полное" {
          }
        }
        n210 = call "AutoScale.vi"("ScaleOrdinate 2"=w269, "Type_signal"=w273, "UNDT_Gain"=w278) -> ("Min"=w262:dbl, "Max"=w263:dbl)  [unwired: 6 in, 1 out]
        n211 = property on="Видеофильтр" class="Bool (strict)"(error in=w266, "DisabledEnum"=w277) -> (error out=w265:errorcluster)  [unwired: 1 in, 1 out]
        n212 = property on="AScanXY" class="XYGraph (strict)"(error in=w265, "YScale.Maximum"=w263, "YScale.Minimum"=w262) -> (error out=w264:errorcluster)  [unwired: 1 in, 1 out]
      }
      event "Connect": Value Change {
        n213 = event-data() -> ()  [unwired: 1 in, 6 out]
        n214 = global read "Global_SNK3_HF.vi" "paramUnicorn"() -> (w292:T9)
        n215 = Unbundle By Name(w292) -> ("conParam.TCP_conn"=w289:bool)
        n216 = Select(t="Disconnect" ("element"), s=w289, f="Connect" ("element")) -> (s? t:f=w288:string)
        n217 = Enqueue Element(queue=w295, element=w288, error in (no error)=w294) -> (queue out=w287:refnum<queue>, error out=w293:errorcluster)  [unwired: 1 in, 1 out]
      }
      event "LPF_Filter": Value Change {
        n218 = event-data() -> ()  [unwired: 1 in, 6 out]
        n219 = call "Msg_NoConEU (SubVI).vi"() -> ("conParam.TCP_conn"=w296:bool)  [unwired: 11 in]
        n220 = case shown="True" w296 {
          tunnel: w300 -> [w302 w307]
          tunnel: w299 -> [w301 w306]
          tunnel: [w301 w305] -> w298
          tunnel: [w302 w303] -> w297
          frame False {
          }
          frame True {
            n221 = Enqueue Element(queue=w307, element="LPF", error in (no error)=w306) -> (queue out=w303:refnum<queue>, error out=w305:errorcluster)  [unwired: 1 in, 1 out]
          }
        }
      }
      event "UNDT_HF_Filter": Value Change {
        n222 = event-data() -> ()  [unwired: 1 in, 6 out]
        n223 = call "Msg_NoConEU (SubVI).vi"() -> ("conParam.TCP_conn"=w308:bool)  [unwired: 11 in]
        n224 = case shown="False" w308 {
          tunnel: w312 -> [w314 w319]
          tunnel: w311 -> [w313 w318]
          tunnel: [w313 w317] -> w310
          tunnel: [w314 w315] -> w309
          frame False {
          }
          frame True {
            n225 = Enqueue Element(queue=w319, element="HPF", error in (no error)=w318) -> (queue out=w315:refnum<queue>, error out=w317:errorcluster)  [unwired: 1 in, 1 out]
          }
        }
      }
      event "UNDT_Start": Value Change {
        n226 = event-data() -> ()  [unwired: 1 in, 6 out]
        n227 = call "Msg_NoConEU (SubVI).vi"() -> ("conParam.TCP_conn"=w320:bool)  [unwired: 11 in]
        n228 = case shown="True" w320 {
          tunnel: w324 -> [w326 w334]
          tunnel: w323 -> [w325 w333]
          tunnel: [w325 w328] -> w322
          tunnel: [w326 w330] -> w321
          frame False {
          }
          frame True {
            n229 = Enqueue Element(queue=w334, element="Start", error in (no error)=w333) -> (queue out=w331:refnum<queue>, error out=w329:errorcluster)  [unwired: 1 in, 1 out]
            n230 = Enqueue Element(queue=w331, element="AutoScaleTime", error in (no error)=w329) -> (queue out=w330:refnum<queue>, error out=w328:errorcluster)  [unwired: 1 in, 1 out]
          }
        }
      }
      event "ScaleAbciss": Value Change {
        n231 = event-data() -> ()  [unwired: 1 in, 6 out]
        n232 = call "Msg_NoConEU (SubVI).vi"() -> ("conParam.TCP_conn"=w339:bool)  [unwired: 11 in]
        n233 = case shown="True" w339 {
          tunnel: w338 -> [w341 w343]
          tunnel: w337 -> [w340 w342]
          tunnel: [w340 w345] -> w335
          tunnel: [w341 w346] -> w336
          frame False {
          }
          frame True {
            n234 = Enqueue Element(queue=w343, element="AutoScaleTime", error in (no error)=w342) -> (queue out=w346:refnum<queue>, error out=w345:errorcluster)  [unwired: 1 in, 1 out]
          }
        }
      }
      event "UNDT_GIV1": Value Change {
        n235 = event-data() -> ()  [unwired: 1 in, 6 out]
        n236 = call "Msg_NoConEU (SubVI).vi"() -> ("conParam.TCP_conn"=w347:bool)  [unwired: 11 in]
        n237 = case shown="True" w347 {
          tunnel: w351 -> [w353 w357]
          tunnel: w350 -> [w352 w356]
          tunnel: [w352 w355] -> w349
          tunnel: [w353 w354] -> w348
          frame False {
          }
          frame True {
            n238 = flat-sequence {
              tunnel: w356 -> [w366]
              tunnel: w357 -> [w367]
              tunnel: [w367] -> w359
              tunnel: [w366] -> w358
              tunnel: [w373] -> w355
              tunnel: w359 -> [w376]
              tunnel: w358 -> [w375]
              tunnel: [w374] -> w354
              frame #0 {
                n239 = global read "Global_SNK3_HF.vi" "TblParam0"() -> (w361:sgl[][])
                n240 = local read "Tick"() -> (w365:i32)
                n241 = local read "WPulse0"() -> (w362:dbl)
                n242 = Decrement(x=w365) -> (x-1=w364:i32)
                n243 = Replace Array Subset(array=w361, new element=w362, index (row)=3 ("disabled index (row)"), index (col)=w364) -> (w360:sgl[][])
                n244 = global write "Global_SNK3_HF.vi" "TblParam0"(w360) -> ()
              }
              frame #1 {
                n245 = Build Array("Stop" ("element"), "GIV1" ("element"), "WrtTable0" ("element"), "Start" ("element")) -> (w368:string[])
                n246 = for {
                  shift-right: [w379] -> w374
                  shift-left: w376 -> [w381]
                  shift-right: [w378] -> w373
                  shift-left: w375 -> [w380]
                  tunnel: w368 -> [w377] mode=indexing
                  n247 = Enqueue Element(queue=w381, element=w377, error in (no error)=w380) -> (queue out=w379:refnum<queue>, error out=w378:errorcluster)  [unwired: 1 in, 1 out]
                }
              }
            }
          }
        }
      }
      event "UNDT_GIV2": Value Change {
        n248 = event-data() -> ()  [unwired: 1 in, 6 out]
        n249 = call "Msg_NoConEU (SubVI).vi"() -> ("conParam.TCP_conn"=w382:bool)  [unwired: 11 in]
        n250 = case shown="True" w382 {
          tunnel: w386 -> [w388 w392]
          tunnel: w385 -> [w387 w391]
          tunnel: [w387 w390] -> w384
          tunnel: [w388 w389] -> w383
          frame False {
          }
          frame True {
            n251 = flat-sequence {
              tunnel: w391 -> [w401]
              tunnel: w392 -> [w402]
              tunnel: [w402] -> w394
              tunnel: [w401] -> w393
              tunnel: [w411] -> w390
              tunnel: w394 -> [w405]
              tunnel: w393 -> [w404]
              tunnel: [w410] -> w389
              frame #0 {
                n252 = global read "Global_SNK3_HF.vi" "TblParam1"() -> (w396:sgl[][])
                n253 = local read "Tick"() -> (w400:i32)
                n254 = local read "PWhite1"() -> (w397:dbl)
                n255 = Decrement(x=w400) -> (x-1=w399:i32)
                n256 = Replace Array Subset(array=w396, new element=w397, index (row)=3 ("disabled index (row)"), index (col)=w399) -> (w395:sgl[][])
                n257 = global write "Global_SNK3_HF.vi" "TblParam1"(w395) -> ()
              }
              frame #1 {
                n258 = Build Array("Stop" ("element"), "GIV2" ("element"), "WrtTable1" ("element"), "Start" ("element")) -> (w403:string[])
                n259 = for {
                  shift-right: [w415] -> w410
                  shift-left: w405 -> [w414]
                  shift-right: [w416] -> w411
                  shift-left: w404 -> [w413]
                  tunnel: w403 -> [w412] mode=indexing
                  n260 = Enqueue Element(queue=w414, element=w412, error in (no error)=w413) -> (queue out=w415:refnum<queue>, error out=w416:errorcluster)  [unwired: 1 in, 1 out]
                }
              }
            }
          }
        }
      }
      event "UNDT_Freq": Value Change {
        n261 = event-data() -> ("OldVal"=w425:i32, "NewVal"=w426:i32)  [unwired: 1 in, 4 out]
        n262 = call "Msg_NoConEU (SubVI).vi"() -> ("conParam.TCP_conn"=w421:bool)  [unwired: 11 in]
        n263 = local read "UNDT_NTick"() -> (w424:i32)
        n264 = call "BandwidthСalc (SubVI).vi"("Freq"=w426, "NTick"=w424) -> ("norm"=w422:bool)  [unwired: 7 in, 2 out]
        n265 = And(x=w421, y=w422) -> (x .and. y?=w420:bool)
        n266 = case shown="True" w420 {
          tunnel: w426 -> [_ w446]
          tunnel: w425 -> [w444 _]
          tunnel: w419 -> [w443 w445]
          tunnel: [w443 w445] -> w418
          frame False {
            n267 = local write "UNDT_Freq"(w444) -> ()
          }
          frame True {
            n268 = local write "UNDT_Freq"(w446) -> ()
          }
        }
        n269 = case shown="True" w420 {
          tunnel: w427 -> [w429 w437]
          tunnel: w418 -> [w428 w436]
          tunnel: [w428 w435] -> w417
          tunnel: [w429 w434] -> w423
          frame False {
          }
          frame True {
            n270 = Build Array("Stop" ("element"), "UNDT_Freq" ("element"), "Start" ("element")) -> (w430:string[])
            n271 = for {
              tunnel: w430 -> [w439] mode=indexing
              shift-right: [w438] -> w434
              shift-left: w437 -> [w442]
              shift-right: [w440] -> w435
              shift-left: w436 -> [w441]
              n272 = Enqueue Element(queue=w442, element=w439, error in (no error)=w441) -> (queue out=w438:refnum<queue>, error out=w440:errorcluster)  [unwired: 1 in, 1 out]
            }
          }
        }
      }
      event "Tick": Value Change {
        n273 = event-data() -> ()  [unwired: 1 in, 6 out]
        n274 = Enqueue Element(queue=w454, element="TickInd", error in (no error)=w453) -> (queue out=w452:refnum<queue>, error out=w451:errorcluster)  [unwired: 1 in, 1 out]
        n275 = Enqueue Element(queue=w452, element="Refresh_AScan", error in (no error)=w451) -> (queue out=w450:refnum<queue>, error out=w449:errorcluster)  [unwired: 1 in, 1 out]
      }
      event "TxDelay0", "RxDelay0", "RxWhite0", "RxCh0", "TxCh0", "WPulse0", "Gain0", "Tx0", "Rx0", "TxPulseCh0": Value Change {
        n276 = event-data() -> ()  [unwired: 1 in, 6 out]
        n277 = flat-sequence {
          tunnel: w471 -> [w485]
          tunnel: [w485] -> w469
          tunnel: [w484] -> w467
          tunnel: w466 -> [w484]
          tunnel: [w483] -> w465
          tunnel: [w508] -> w470
          tunnel: w469 -> [w508]
          tunnel: [w507] -> w468
          tunnel: w467 -> [w507]
          tunnel: w465 -> [w506]
          frame #0 {
            n278 = local read "Tick"() -> (w482:i32)
            n279 = Boolean To (0,1)(Boolean="Tx0") -> (0, 1=w504:i16)
            n280 = global read "Global_SNK3_HF.vi" "TblParam0"() -> (w483:sgl[][])
            n281 = To Double Precision Float(number=w504) -> (double precision float=w495:dbl)
            n282 = Boolean To (0,1)(Boolean="Rx0") -> (0, 1=w503:i16)
            n283 = To Double Precision Float(number="RxCh0") -> (double precision float=w500:dbl)
            n284 = To Double Precision Float(number="TxPulseCh0") -> (double precision float=w478:dbl)
            n285 = To Double Precision Float(number="TxCh0") -> (double precision float=w496:dbl)
            n286 = To Double Precision Float(number=w503) -> (double precision float=w499:dbl)
            n287 = Number To Decimal String(number="RxCh0") -> (decimal integer string=w492:string)  [unwired: 1 in]
            n288 = Decrement(x=w482) -> (x-1=w488:i32)
            n289 = Build Array(w495, w496, "TxDelay0", "WPulse0", w499, w500, "RxDelay0", "RxWhite0", "Gain0", 0.0 ("element"), w478) -> (w494:dbl[])
            n290 = control-ref of="AScanXY"() -> (w477:refnum<vi>)
            n291 = Replace Array Subset(array=w483, new element=w494, index (col)=w488) -> (w486:sgl[][])  [unwired: 1 in]
            n292 = Build Array(w477) -> (w481:refnum<vi>[])
            n293 = global write "Global_SNK3_HF.vi" "TblParam0"(w486) -> ()
            n294 = call "Graph_legend (SubVI).vi"("Numeric"=w488, "rb"=0, "String"=w492, "appended array"=w481) -> ()  [unwired: 8 in]
          }
          frame #1 {
            n295 = local read "UNDT_NTick"() -> (w511:i32)
            n296 = local read "UNDT_Freq"() -> (w510:i32)
            n297 = call "BandwidthСalc (SubVI).vi"("Freq"=w510, "NTick"=w511) -> ("norm"=w509:bool)  [unwired: 7 in, 2 out]
            n298 = case shown="False" w509 {
              tunnel: w506 -> [w512 _]
              frame False {
                n299 = global write "Global_SNK3_HF.vi" "TblParam0"(w512) -> ()
              }
              frame True {
              }
            }
          }
        }
        n300 = Build Array("Stop" ("element"), "WrtTable0" ("element"), "AutoScaleTime" ("element"), "AutoScale" ("element"), "Refresh_AScan" ("element"), "TickInd" ("element"), "Start" ("element")) -> (w459:string[])
        n301 = for {
          shift-right: [w474] -> w461
          shift-left: w470 -> [w476]
          shift-right: [w473] -> w460
          shift-left: w468 -> [w475]
          tunnel: w459 -> [w472] mode=indexing
          n302 = Enqueue Element(queue=w475, element=w472, error in (no error)=w476) -> (queue out=w473:refnum<queue>, error out=w474:errorcluster)  [unwired: 1 in, 1 out]
        }
      }
      event "Tx1", "Rx1", "TxCh1", "RxCh1", "TxDelay1", "PWhite1", "RxDelay1", "RxWhite1", "Gain1", "TxPulseCh1": Value Change {
        n303 = event-data() -> ()  [unwired: 1 in, 6 out]
        n304 = flat-sequence {
          tunnel: w529 -> [w557]
          tunnel: [w557] -> w528
          tunnel: w527 -> [w556]
          tunnel: [w556] -> w526
          tunnel: [w541] -> w525
          tunnel: w528 -> [w569]
          tunnel: w526 -> [w568]
          tunnel: [w569] -> w520
          tunnel: [w568] -> w519
          tunnel: w525 -> [w564]
          frame #0 {
            n305 = global read "Global_SNK3_HF.vi" "TblParam1"() -> (w541:sgl[][])
            n306 = local read "Tick"() -> (w540:i32)
            n307 = To Double Precision Float(number="TxCh1") -> (double precision float=w559:dbl)
            n308 = To Double Precision Float(number="TxPulseCh1") -> (double precision float=w536:dbl)
            n309 = Boolean To (0,1)(Boolean="Tx1") -> (0, 1=w563:i16)
            n310 = Decrement(x=w540) -> (x-1=w543:i32)
            n311 = Boolean To (0,1)(Boolean="Rx1") -> (0, 1=w562:i16)
            n312 = control-ref of="AScanXY"() -> (w535:refnum<vi>)
            n313 = To Double Precision Float(number="RxCh1") -> (double precision float=w561:dbl)
            n314 = To Double Precision Float(number=w563) -> (double precision float=w558:dbl)
            n315 = To Double Precision Float(number=w562) -> (double precision float=w560:dbl)
            n316 = Number To Decimal String(number="RxCh1") -> (decimal integer string=w548:string)  [unwired: 1 in]
            n317 = Build Array(w558, w559, "TxDelay1", "PWhite1", w560, w561, "RxDelay1", "RxWhite1", "Gain1", 0.0 ("element"), w536) -> (w555:dbl[])
            n318 = Replace Array Subset(array=w541, new element=w555, index (col)=w543) -> (w544:sgl[][])  [unwired: 1 in]
            n319 = Build Array(w535) -> (w539:refnum<vi>[])
            n320 = global write "Global_SNK3_HF.vi" "TblParam1"(w544) -> ()
            n321 = call "Graph_legend (SubVI).vi"("Numeric"=w543, "rb"=1, "String"=w548, "appended array"=w539) -> ()  [unwired: 8 in]
          }
          frame #1 {
            n322 = local read "UNDT_NTick"() -> (w566:i32)
            n323 = local read "UNDT_Freq"() -> (w567:i32)
            n324 = call "BandwidthСalc (SubVI).vi"("Freq"=w567, "NTick"=w566) -> ("norm"=w565:bool)  [unwired: 7 in, 2 out]
            n325 = case shown="False" w565 {
              tunnel: w564 -> [w570 _]
              frame False {
                n326 = global write "Global_SNK3_HF.vi" "TblParam1"(w570) -> ()
              }
              frame True {
              }
            }
          }
        }
        n327 = Build Array("Stop" ("element"), "WrtTable1" ("element"), "AutoScaleTime" ("element"), "AutoScale" ("element"), "Refresh_AScan" ("element"), "TickInd" ("element"), "Start" ("element")) -> (w521:string[])
        n328 = for {
          shift-right: [w532] -> w518
          shift-left: w519 -> [w534]
          shift-right: [w531] -> w517
          shift-left: w520 -> [w533]
          tunnel: w521 -> [w530] mode=indexing
          n329 = Enqueue Element(queue=w533, element=w530, error in (no error)=w534) -> (queue out=w531:refnum<queue>, error out=w532:errorcluster)  [unwired: 1 in, 1 out]
        }
      }
      event "RingMenu": Value Change {
        n330 = event-data() -> ()  [unwired: 1 in, 6 out]
        n331 = local write "TabRight"("RingMenu") -> ()
      }
      event "UNDT_NTick": Value Change {
        n332 = event-data() -> ("OldVal"=w576:i32, "NewVal"=w577:i32)  [unwired: 1 in, 4 out]
        n333 = call "Msg_NoConEU (SubVI).vi"() -> ("conParam.TCP_conn"=w574:bool)  [unwired: 11 in]
        n334 = case shown="True" w574 {
          tunnel: w580 -> [w581 w588]
          tunnel: w579 -> [w582 w592]
          tunnel: [w582 w590] -> w578
          tunnel: w577 -> [_ w596]
          tunnel: w576 -> [_ w593]
          tunnel: [w581 w591] -> w575
          frame False {
          }
          frame True {
            n335 = flat-sequence {
              tunnel: [w605] -> w597
              tunnel: w596 -> [w604]
              tunnel: [w604] -> w595
              tunnel: [w603] -> w594
              tunnel: w593 -> [w603]
              tunnel: w597 -> [w609]
              tunnel: w595 -> [w608]
              tunnel: w594 -> [w607]
              tunnel: [w613] -> w589
              tunnel: w592 -> [w613]
              frame #0 {
                n336 = local read "UNDT_Freq"() -> (w606:i32)
                n337 = call "BandwidthСalc (SubVI).vi"("Freq"=w606, "NTick"=w604) -> ("norm"=w605:bool)  [unwired: 7 in, 2 out]
              }
              frame #1 {
                n338 = case shown="True" w609 {
                  tunnel: w608 -> [_ w611]
                  tunnel: w607 -> [w610 _]
                  frame False {
                    n339 = local write "UNDT_NTick"(w610) -> ()
                  }
                  frame True {
                    n340 = local write "UNDT_NTick"(w611) -> ()
                  }
                }
              }
              frame #2 {
                n341 = Wait (ms)(milliseconds to wait=u32 100) -> ()  [unwired: 1 out]
                n342 = local read "ScaleOrdinate"() -> (w615:T4)
                n343 = call "TableCollum(SubVI).vi"("ScaleOrdinate 2"=w615, "UNDT_NTick"=1) -> ("array"=w614:string[][])  [unwired: 9 in]
                n344 = local write "UNDT_meas"(w614) -> ()
              }
            }
            n345 = Build Array("Stop" ("element"), "NTick" ("element"), "Refresh_AScan" ("element"), "Start" ("element")) -> (w583:string[])
            n346 = for {
              shift-right: [w601] -> w590
              shift-left: w589 -> [w600]
              shift-right: [w602] -> w591
              shift-left: w588 -> [w599]
              tunnel: w583 -> [w598] mode=indexing
              n347 = Enqueue Element(queue=w599, element=w598, error in (no error)=w600) -> (queue out=w602:refnum<queue>, error out=w601:errorcluster)  [unwired: 1 in, 1 out]
            }
          }
        }
      }
      event "Save": Value Change {
        n348 = event-data() -> ()  [unwired: 1 in, 6 out]
        n349 = invoke on="AScanXY" class="XYGraph (strict)" method="Export Data to Excel"(error in=w618) -> (error out=w617:errorcluster)  [unwired: 2 in, 2 out]
      }
      event Menu Selection (User) {
        n350 = event-data() -> ("ItemTag"=w624:string)  [unwired: 1 in, 6 out]
        n351 = case shown="\"parameters_EU\"" w624 {
          tunnel: [w626 w627 w633 w645 w648 w650 w654 w658 w662 w665 w668 w673] -> w623
          tunnel: w622 -> [w626 w627 w634 w645 w648 w650 w654 w658 w662 w665 w668 w673]
          tunnel: w621 -> [w625 w628 w631 w646 w647 w651 w653 w657 w661 w666 w669 w672]
          tunnel: [w625 w628 w632 w646 w647 w651 w653 w657 w661 w666 w669 w672] -> w620
          frame "False", Default {
          }
          frame "About" {
            n352 = global read "Global_SNK3_HF.vi" "About_prg"() -> (w629:T21)
            n353 = call "Dialog_about_program (SubVI).vi"("Param"=w629) -> ()  [unwired: 11 in]
          }
          frame "tblParam" {
            n354 = call "Msg_NoConEU (SubVI).vi"() -> ("conParam.TCP_conn"=w630:bool)  [unwired: 11 in]
            n355 = case shown="True" w630 {
              tunnel: w634 -> [w636 w643]
              tunnel: [w636 w642] -> w633
              tunnel: [w635 w640] -> w632
              tunnel: w631 -> [w635 w639]
              frame False {
              }
              frame True {
                n356 = control-ref of="Log"() -> (w637:refnum<vi>)
                n357 = call "ParametersTable.vi"("error in (no error)"=w639, "Log"=w637) -> ("error out"=w638:errorcluster)  [unwired: 8 in, 1 out]
                n358 = Enqueue Element(queue=w643, element="TickInd", error in (no error)=w638) -> (queue out=w642:refnum<queue>, error out=w640:errorcluster)  [unwired: 1 in, 1 out]
              }
            }
          }
          frame "Debug" {
            n359 = vi-ref "Dialog_debug (SubVI).vi"() -> ()  [unwired: 1 out]
            n360 = vi-ref "Global_SNK3_HF.vi"() -> (w644:refnum<vi>)
            n361 = call "RunVI (SubVI).vi"("VI in"=w644) -> ()  [unwired: 11 in]
          }
          frame "Reset_stat_UNDT" {
            n362 = call "ResetStat.vi"() -> ()  [unwired: 12 in]
          }
          frame "TestGIV" {
            n363 = call "Msg_NoConEU (SubVI).vi"() -> ("conParam.TCP_conn"=w649:bool)  [unwired: 11 in]
            n364 = case shown="True" w649 {
              frame False {
              }
              frame True {
                n365 = vi-ref "Dialog_TestGIV (SubVI).vi"() -> (w652:refnum<vi>)
                n366 = call "RunVI (SubVI).vi"("VI in"=w652) -> ()  [unwired: 11 in]
              }
            }
          }
          frame "Spectr" {
            n367 = vi-ref "Dialog_Spectr2 (SubVI).vi"() -> (w655:refnum<vi>)
            n368 = call "RunVI (SubVI).vi"("VI in"=w655) -> ()  [unwired: 11 in]
          }
          frame "TestRB" {
            n369 = call "Msg_NoConEU (SubVI).vi"() -> ("conParam.TCP_conn"=w656:bool)  [unwired: 11 in]
            n370 = case shown="True" w656 {
              frame False {
              }
              frame True {
                n371 = vi-ref "Dialog_TestGC (SubVI).vi"() -> (w659:refnum<vi>)
                n372 = call "RunVI (SubVI).vi"("VI in"=w659) -> ()  [unwired: 11 in]
              }
            }
          }
          frame "TestRBBode" {
            n373 = call "Msg_NoConEU (SubVI).vi"() -> ("conParam.TCP_conn"=w660:bool)  [unwired: 11 in]
            n374 = case shown="True" w660 {
              frame False {
              }
              frame True {
                n375 = vi-ref "Dialog_TestBode (SubVI).vi"() -> (w663:refnum<vi>)
                n376 = call "RunVI (SubVI).vi"("VI in"=w663) -> ()  [unwired: 11 in]
              }
            }
          }
          frame "MeasureLog" {
            n377 = call "Msg_NoConEU (SubVI).vi"() -> ("conParam.TCP_conn"=w664:bool)  [unwired: 11 in]
            n378 = case shown="True" w664 {
              frame False {
              }
              frame True {
                n379 = vi-ref "Dialog_LogMeas (SubVI).vi"() -> (w667:refnum<vi>)
                n380 = call "RunVI (SubVI).vi"("VI in"=w667) -> ()  [unwired: 11 in]
              }
            }
          }
          frame "parameters_EU" {
            n381 = stacked-sequence {
              frame #0 {
                n382 = call "Msg_NoConEU (SubVI).vi"() -> ("conParam.TCP_conn"=w670:bool)  [unwired: 11 in]
                n383 = case shown="True" w670 {
                  frame False {
                  }
                  frame True {
                    n384 = call "Dialog_parameters (SubVI).vi"() -> ()  [unwired: 11 in, 1 out]
                  }
                }
              }
              frame #1 {
                n385 = control-ref of="Table"() -> (w671:refnum<vi>)
                n386 = call "String_Indicator (SubVI).vi"("String in"=w671) -> ()  [unwired: 11 in]
              }
            }
          }
          frame "True" {
          }
        }
      }
      event "ScaleOrdinate": Value Change {
        n387 = event-data() -> ("NewVal"=w676:T4)  [unwired: 1 in, 5 out]
        n388 = global read "Global_SNK3_HF.vi" "OptPACKPL0"() -> (w681:T23)
        n389 = global read "Global_SNK3_HF.vi" "OptPACKPL1"() -> (w677:T23)
        n390 = Bundle By Name(cluster=w681, "ScaleOrdinate"=w676) -> (w680:T23)
        n391 = Bundle By Name(cluster=w677, "ScaleOrdinate"=w676) -> (w678:T23)
        n392 = global write "Global_SNK3_HF.vi" "OptPACKPL0"(w680) -> ()
        n393 = global write "Global_SNK3_HF.vi" "OptPACKPL1"(w678) -> ()
        n394 = case shown="\"Отсчеты АЦП (±32767)\", Default" "ScaleOrdinate" {
          tunnel: [FALSE ("DataTo1") TRUE ("DataTo1") TRUE ("DataTo1") TRUE ("DataTo1")] -> _
          tunnel: [FALSE ("DataTo1") FALSE ("DataTo1") TRUE ("DataTo1") TRUE ("DataTo1")] -> _
          frame "Отсчеты АЦП (±32767)", Default {
            n395 = local read "ScaleADC"() -> (w687:bool)
            n396 = case shown="True" w687 {
              frame False {
              }
              frame True {
                n397 = local write "ScaleADC"(FALSE ("ScaleADC")) -> ()
              }
            }
          }
          frame "Проценты" {
            n398 = local write "ScaleADC"(TRUE ("ScaleADC")) -> ()
          }
          frame "Вольты" {
            n399 = local write "ScaleADC"(TRUE ("ScaleADC")) -> ()
          }
          frame "дБмкВ (отн. 1 мкВ)" {
            n400 = local read "Type_signal"() -> (w699:T7)
            n401 = Equal?(x=w699, y=T7."РЧ сигнал" ("Type_signal")) -> (x = y?=w697:bool)
            n402 = case shown="True" w697 {
              frame False {
              }
              frame True {
                n403 = local write "Type_signal"(T7."Детект. полное" ("Type_signal")) -> ()
              }
            }
          }
        }
        n404 = call "TableCollum(SubVI).vi"("ScaleOrdinate 2"="ScaleOrdinate", "UNDT_NTick"=1) -> ("array"=w682:string[][])  [unwired: 9 in]
        n405 = local write "UNDT_meas"(w682) -> ()
        n406 = Enqueue Element(queue=w686, element="ScaleOrdinate", error in (no error)=w684) -> (queue out=w679:refnum<queue>, error out=w683:errorcluster)  [unwired: 1 in, 1 out]
      }
      event Panel Close? {
        n407 = event-data() -> ()  [unwired: 1 in, 4 out]
        n408 = disable-structure shown="Enabled" {
          disable-tunnel: [w711 w712] -> w704
          disable-tunnel: w703 -> [w708 w712]
          frame Enabled {
            n409 = control-ref of="Log"() -> (w710:refnum<vi>)
            n410 = call "LogAdd (SubVI).vi"("error in"=w708, "string"="Закрытие ПО", "Log"=w710) -> ("error out"=w707:errorcluster)  [unwired: 8 in]
            n411 = call <vilib>:"Clear Errors.vi"("error in (no error)"=w707) -> ("error out"=w711:errorcluster)  [unwired: 5 in, 1 out]
          }
          frame Disabled {
          }
        }
        n412 = global write "Global_SNK3_HF.vi" "Stop"(TRUE ("Stop")) -> ()
        n413 = event-data() -> ()  [unwired: 2 in, 1 out]
      }
      event "AutoScaleTime": Value Change {
        n414 = event-data() -> ()  [unwired: 1 in, 6 out]
        n415 = Enqueue Element(queue=w717, element="AutoScaleTime", error in (no error)=w716) -> (queue out=w713:refnum<queue>, error out=w715:errorcluster)  [unwired: 1 in, 1 out]
      }
      event "SaveParam": Value Change {
        n416 = event-data() -> ()  [unwired: 1 in, 6 out]
        n417 = local read "Connect"() -> (w719:bool)
        n418 = case shown="True" w719 {
          tunnel: w722 -> [w723 w729]
          tunnel: w721 -> [w724 w728]
          tunnel: [w724 w727] -> w720
          tunnel: [w723 w725] -> w718
          frame False {
          }
          frame True {
            n419 = Enqueue Element(queue=w729, element="SaveParam", error in (no error)=w728) -> (queue out=w725:refnum<queue>, error out=w727:errorcluster)  [unwired: 1 in, 1 out]
          }
        }
      }
      event Mouse Wheel {
        n420 = event-data() -> ("CtlRef"=w738:refnum<vi>, "Delta"=w737:i32)  [unwired: 1 in, 4 out]
        n421 = local read "ScaleOrdinate"() -> (w736:T4)
        n422 = property on="Property Node" class="XYGraph (strict)"(reference=w738, error in=w731) -> (reference out=w741:refnum<vi>, error out=w732:errorcluster, "YScale.Range"=w733:T27)
        n423 = case shown="\"Вольты\"" w736 {
          tunnel: [cluster{"max":dbl, "increment":dbl} {"max"=32767.0, "increment"=250.0} ("Param") w749 cluster{"max":dbl, "increment":dbl} {"max"=140.0, "increment"=1.0} ("Param") cluster{"max":dbl, "increment":dbl} {"max"=1.2, "increment"=0.05} ("Param") cluster{"max":dbl, "increment":dbl} {"max"=100.0, "increment"=5.0} ("Param")] -> w735
          tunnel: w733 -> [_ w748 _ _ _]
          frame "Отсчеты АЦП (±32767)", Default {
          }
          frame "Вольты" {
            n424 = Unbundle By Name(w748) -> ("Maximum"=w744:dbl)
            n425 = Greater?(x=w744, y=0.05) -> (0:w746:bool)
            n426 = Greater?(x=w744, y=0.001) -> (0:w743:bool)
            n427 = case shown="False" w746 {
              tunnel: [w751 cluster{"max":dbl, "increment":dbl} {"max"=1.4, "increment"=0.025} ("Param")] -> w749
              tunnel: w743 -> [w750 _]
              frame False {
                n428 = case shown="False" w750 {
                  tunnel: [cluster{"max":dbl, "increment":dbl} {"max"=1.4, "increment"=0.0002} ("Param") cluster{"max":dbl, "increment":dbl} {"max"=1.4, "increment"=0.001} ("Param")] -> w751
                  frame False {
                  }
                  frame True {
                  }
                }
              }
              frame True {
              }
            }
          }
          frame "дБмкВ (отн. 1 мкВ)" {
          }
          frame "Отсчеты АЦП (±1)" {
          }
          frame "Проценты" {
          }
        }
        n429 = call "Zoom_graph (SubVI).vi"("Delta"=w737, "Param"=w735, "YScale.Range in"=w733) -> ("Boolean"=w740:bool, "YScale.Range out"=w739:T27)  [unwired: 7 in]
        n430 = case shown="True" w740 {
          tunnel: w739 -> [_ w764]
          tunnel: w741 -> [_ w763]
          tunnel: w732 -> [w758 w760]
          tunnel: [w758 w759] -> w730
          frame False {
          }
          frame True {
            n431 = local read "Type_signal"() -> (w762:T7)
            n432 = case shown="\"Детект. полное\"" w762 {
              tunnel: w764 -> [w765 w768 w770 w773]
              tunnel: w763 -> [_ _ _ _]
              tunnel: [w765 w766 w769 w772] -> w761
              frame "РЧ сигнал", Default {
              }
              frame "Детект. полное" {
                n433 = Bundle By Name(cluster=w768, "Minimum"=0.0) -> (w766:T27)
              }
              frame "Положит." {
                n434 = Bundle By Name(cluster=w770, "Minimum"=0.0) -> (w769:T27)
              }
              frame "Отрицат." {
                n435 = Bundle By Name(cluster=w773, "Minimum"=0.0) -> (w772:T27)
              }
            }
            n436 = property on="Property Node" class="XYGraph (strict)"(reference=w763, error in=w760, "YScale.Range"=w761) -> (error out=w759:errorcluster)  [unwired: 1 out]
          }
        }
      }
      event "save_osc": Value Change {
        n437 = event-data() -> ("OldVal"=w778:bool[], "NewVal"=w777:bool[])  [unwired: 1 in, 4 out]
        n438 = for {
          tunnel: w778 -> [w782] mode=indexing
          tunnel: w777 -> [w779] mode=indexing
          i -> [w780]
          n439 = Not Equal?(x=w782, y=w779) -> (x != y?=w781:bool)
          n440 = case shown="True" w781 {
            tunnel: w780 -> [_ w787]
            tunnel: w779 -> [_ w783]
            frame False {
            }
            frame True {
              n441 = local read "AScanXY"() -> (w788:T1)
              n442 = Add(x=64, y=w787) -> (x+y=w785:i32)
              n443 = case shown="False" w783 {
                tunnel: w788 -> [w792 w797]
                tunnel: w785 -> [w790 w794]
                tunnel: [w791 w793] -> w784
                frame False {
                  n444 = Replace Array Subset(array=w792, new element=cluster{dbl[], dbl[]} {[], []} ("XY Graph"), index=w790) -> (w791:T1)
                }
                frame True {
                  n445 = Index Array(array=w797, index="index_osc") -> (element=w795:cluster{dbl[], dbl[]})
                  n446 = Replace Array Subset(array=w797, new element=w795, index=w794) -> (w793:T1)
                }
              }
              n447 = local write "AScanXY"(w784) -> ()
            }
          }
        }
      }
      event "Refresh": Value Change {
        n448 = event-data() -> ()  [unwired: 1 in, 6 out]
        n449 = Enqueue Element(queue=w802, element="Refresh_AScan", error in (no error)=w801) -> (queue out=w798:refnum<queue>, error out=w799:errorcluster)  [unwired: 1 in, 1 out]
      }
      event Panel Resize {
        w831 = T26 {"Width"=1543, "Height"=895} ("Plot Area:Size 2")
        n450 = event-data() -> ("NewBnds"=w842:T28)  [unwired: 1 in, 7 out]
        n451 = Unbundle By Name(w842) -> ("Top"=w840:i16, "Bottom"=w841:i16, "Left"=w835:i16, "Right"=w836:i16)
        n452 = Subtract(x=w841, y=w840) -> (x-y=w833:i16)
        n453 = Subtract(x=w836, y=w835) -> (x-y=w834:i16)
        n454 = Subtract(x=w833, y=u32 824 ("x")) -> (x-y=w838:u32)
        n455 = Add(x=u32 36, y=w838) -> (x+y=w815:u32)
        n456 = property on="Log" class="Str"("Height"=w815) -> ()  [unwired: 2 in, 2 out]
        n457 = Bundle By Name(cluster=w831, "Width"=w834, "Height"=w833) -> (w832:T26)
        n458 = Subtract(x=w832, y=w831) -> (x-y=w806:T26)
        n459 = Add(x=T26 {"Width"=815, "Height"=860} ("Plot Area:Size 2"), y=w806) -> (x+y=w818:T26)
        n460 = Add(x=T25 {"Left"=932, "Top"=618} ("Position"), y=w806) -> (x+y=w827:T26)
        n461 = Add(x=T25 {"Left"=938, "Top"=585} ("Position"), y=w806) -> (x+y=w825:T26)
        n462 = property on="AScanXY" class="XYGraph (strict)"(error in=w823, "Position"=T25 {"Left"=0, "Top"=-40}) -> (error out=w817:errorcluster)  [unwired: 1 in, 1 out]
        n463 = Add(x=T25 {"Left"=938, "Top"=558} ("Position"), y=w806) -> (x+y=w819:T26)
        n464 = property on="AScanXY" class="XYGraph (strict)"(error in=w817, "Plot Area Size"=w818) -> (error out=w816:errorcluster)  [unwired: 1 in, 1 out]
        n465 = property on="UNDT_meas" class="Tbl (strict)"(error in=w816, "Position"=w827) -> (error out=w824:errorcluster)  [unwired: 1 in, 1 out]
        n466 = property on="FreqFind" class="DigNum (strict)"(error in=w824, "Position"=w825) -> (error out=w821:errorcluster)  [unwired: 1 in, 1 out]
        n467 = property on="ScaleOrdinate" class="Enum (strict)"(error in=w821, "Position"=w819) -> (error out=w814:errorcluster)  [unwired: 1 in, 1 out]
        n468 = Add(x=T25 {"Left"=938, "Top"=483} ("Position"), y=w806) -> (x+y=w810:T26)
        n469 = property on="ScaleAbciss" class="Enum (strict)"(error in=w814, "Position"=w810) -> (error out=w813:errorcluster)  [unwired: 1 in, 1 out]
        n470 = Add(x=T25 {"Left"=938, "Top"=456} ("Position 2"), y=w806) -> (x+y=w809:T26)
        n471 = property on="AutoScaleTime" class="Bool (strict)"(error in=w813, "Position"=w809) -> (error out=w808:errorcluster)  [unwired: 1 in, 1 out]
        n472 = Unbundle By Name(w806) -> ("Width"=w804:u32)
        n473 = Add(x=1125 ("Left"), y=w804) -> (x+y=w803:u32)
        n474 = property on="Overload" class="Arr"(error in=w808, "Left"=w803) -> (error out=w807:errorcluster)  [unwired: 1 in, 1 out]
      }
      event "Ind": Value Change {
        n475 = event-data() -> ()  [unwired: 1 in, 6 out]
        n476 = global write "Global_SNK3_HF.vi" "Ind"("Ind") -> ()
      }
    }
    n477 = Unbundle By Name(w218) -> ("status"=w220:bool)
    n478 = Or(x=w220, y=w219) -> (x .or. y?=w217:bool)
  }
  n479 = while {
    tunnel: w4 -> [w850]
    tunnel: w2 -> [w847]
    stop <- w848 stop-if-true
    n480 = Dequeue Element(queue=w850, error in (no error)=w847) -> (element=w846:string, error out=w849:errorcluster)  [unwired: 1 in, 2 out]
    n481 = case shown="No Error" w849 {
      selector: w849 -> [w853 _]
      tunnel: w846 -> [w854 _]
      tunnel: [_ TRUE] -> w848
      frame No Error {
        w851 = T18 1 items=["no dialog", "OK message", "continue or stop message", "OK message + warnings", "continue/stop + warnings"] ("type of dialog (OK msg:1)")
        n482 = case shown="\"Connect\"" w854 {
          tunnel: w853 -> [w855 w864 _ w947 _ w1001 w1009 w1011 w1015 w1018 w1020 w1024 w1028 w1032 w1035 w1038 w1042 w1045 w1049 w1053 w1060 w1071 w1082 w1092]
          tunnel: [w855 w865 w891 w948 w971 w1000 w1009 w1010 w1014 w1018 w1019 w1023 w1027 w1031 w1034 w1037 w1041 w1044 w1048 w1052 w1058 w1069 w1080 w1091] -> w852
          frame "AutoScale" {
            n483 = case shown="True" FALSE {
              frame False {
              }
              frame True {
                n484 = local read "ScaleOrdinate"() -> (w859:T4)
                n485 = local read "Type_signal"() -> (w863:T7)
                n486 = local read "Gain0"() -> (w862:dbl)
                n487 = local read "Gain1"() -> (w861:dbl)
                n488 = Max & Min(x=w862, y=w861) -> (min(x,y)=w860:dbl)  [unwired: 1 out]
                n489 = call "AutoScale.vi"("ScaleOrdinate 2"=w859, "Type_signal"=w863, "UNDT_Gain"=w860) -> ("Min"=w857:dbl, "Max"=w858:dbl)  [unwired: 6 in, 1 out]
                n490 = property on="AScanXY" class="XYGraph (strict)"("YScale.Maximum"=w858, "YScale.Minimum"=w857) -> ()  [unwired: 2 in, 2 out]
              }
            }
          }
          frame "AutoScaleTime" {
            n491 = local read "AutoScaleTime"() -> (w868:bool)
            n492 = case shown="True" w868 {
              tunnel: [w869 "Выключен авто массштаб оси абсцисс (времени)" ("string")] -> w866
              frame True {
                n493 = case shown="True" TRUE {
                  tunnel: ["" ("string") "Включен авто массштаб оси абсцисс (времени)" ("string")] -> w869
                  frame False {
                  }
                  frame True {
                    n494 = global read "Global_SNK3_HF.vi" "TblParam1"() -> (w874:sgl[][])
                    n495 = global read "Global_SNK3_HF.vi" "TblParam0"() -> (w875:sgl[][])
                    n496 = local read "UNDT_NTick"() -> (w880:i32)
                    n497 = local read "ScaleAbciss"() -> (w877:enum16{"Время", "Растояние"})
                    n498 = call "AutoScaleTime (SubVI).vi"("Numeric 3"=w880, "TblPrm2"=w874, "TableParam 0"=w875) -> ("Numeric 2"=w879:sgl, "Numeric"=w878:sgl)  [unwired: 7 in]
                    n499 = case shown="\"Растояние\"" w877 {
                      tunnel: w879 -> [w881 w889]
                      tunnel: [w881 w886] -> w872
                      tunnel: w878 -> [w882 w884]
                      tunnel: [w882 w883] -> w873
                      frame "Время", Default {
                      }
                      frame "Растояние" {
                        n500 = local read "speed"() -> (w888:dbl)
                        n501 = Divide(x=w888, y=2.0) -> (x/y=w885:dbl)
                        n502 = Multiply(x=w889, y=w885) -> (x*y=w886:dbl)
                        n503 = Multiply(x=w884, y=w885) -> (x*y=w883:dbl)
                      }
                    }
                    n504 = property on="AScanXY" class="XYGraph (strict)"("XScale.Maximum"=w873, "XScale.Minimum"=w872) -> ()  [unwired: 2 in, 2 out]
                  }
                }
              }
              frame False {
              }
            }
            n505 = control-ref of="Log"() -> (w867:refnum<vi>)
            n506 = call "LogAdd (SubVI).vi"("error in"=w864, "string"=w866, "Log"=w867) -> ("error out"=w865:errorcluster)  [unwired: 8 in]
          }
          frame "Connect" {
            n507 = control-ref of="Log"() -> (w894:refnum<vi>)
            n508 = call "FindSNK3 (SubVI).vi"("String in"=w894) -> ("error out"=w895:errorcluster, "Cancel"=w893:bool)  [unwired: 9 in]
            n509 = case shown="False" w893 {
              tunnel: w895 -> [w900 w945]
              tunnel: w894 -> [w897 _]
              tunnel: [w898 FALSE ("conParam.TCP_conn")] -> w892
              tunnel: [w896 w945] -> w891
              frame False {
                n510 = call "ConnSNK3 (SubVI).vi"("error in (no error)"=w900, "String in"=w897) -> ("error out"=w899:errorcluster, "conParam.TCP_conn"=w898:bool)  [unwired: 8 in]
                n511 = case shown="True" w898 {
                  tunnel: w899 -> [w901 w905]
                  tunnel: w897 -> [_ w911]
                  tunnel: [w901 w902] -> w896
                  frame False {
                  }
                  frame True {
                    n512 = stacked-sequence {
                      tunnel: w905 -> [w914 _ _ _]
                      tunnel: w911 -> [w913 _ _ _]
                      tunnel: [w912 _ _ _] -> w904
                      frame #0 {
                        w923 = 1 ("UNDT_NTick")
                        w922 = 25 ("Freq")
                        w926 = TRUE ("FPGA0ExtRAMBuffEn")
                        n513 = global read "Global_SNK3_HF.vi" "IP_PC"() -> (w927:string)
                        n514 = call "12_UNDT_IPAddressUDP (SubVI).vi"("error in"=w914, "IP_PC"=w927, "String in"=w913) -> ("error out"=w921:errorcluster)  [unwired: 8 in]
                        n515 = local write "UNDT_Freq"(w922) -> ()
                        n516 = call "24_UNDT_Freq (SubVI).vi"("error in"=w921, "UNDT_Freq"=w922, "String in"=w913) -> ("error out"=w920:errorcluster)  [unwired: 8 in]
                        n517 = call "02_UNDT_CCTicksCount (SubVI).vi"("error in"=w920, "UNDT_NTick"=w923, "String in"=w913) -> ("error out"=w919:errorcluster)  [unwired: 8 in]
                        n518 = local write "UNDT_NTick"(w923) -> ()
                        n519 = call "63_UNDT_FPGA0ExtRAMBuffEn (SubVI).vi"("error in"=w919, "FPGA0ExtRAMBuffEn"=w926, "String in"=w913) -> ("error out"=w925:errorcluster)  [unwired: 7 in, 1 out]
                        n520 = local read "Tick"() -> (w918:i32)
                        n521 = local read "UNDT_HF_Filter"() -> (w917:u16)
                        n522 = call "64_UNDT_FPGA1ExtRAMBuffEn (SubVI).vi"("error in"=w925, "FPGA1ExtRAMBuffEn"=w926, "String in"=w913) -> ("error out"=w924:errorcluster)  [unwired: 8 in]
                        n523 = call "54_UNDT_setKp_dB (SubVI).vi"("error in"=w924, "String in"=w913) -> ("error out"=w916:errorcluster)  [unwired: 9 in]
                        n524 = call "04_UNDT_HPFilter (SubVI).vi"("error in"=w916, "UNDT_HF_Filter"=w917, "String in"=w913) -> ("error out"=w915:errorcluster)  [unwired: 8 in]
                        n525 = call "TickInd (SubVI).vi"("error in (no error)"=w915, "Tick"=w918) -> ("error out"=w912:errorcluster)  [unwired: 9 in]
                      }
                      frame #1 {
                        n526 = global read "Global_SNK3_HF.vi" "ArrayInt"() -> (w928:i32[])
                        n527 = Index Array(array=w928, index #1=1 ("index"), index #2=2 ("index"), index #3=3 ("index"), index #4=4 ("index"), index #5=6 ("index"), index #6=7 ("index")) -> (element #1=w936:i32, element #3=w940:i32, element #4=w939:i32, element #5=w938:i32, element #6=w937:i32)  [unwired: 1 out]
                        n528 = Greater Than 0?(x=w936) -> (x > 0?=w935:bool)
                        n529 = local write "UNDT_HF_Filter"(w939) -> ()
                        n530 = local write "UNDT_GIV1"(w938) -> ()
                        n531 = local write "UNDT_GIV2"(w937) -> ()
                        n532 = local write "UNDT_Start"(w935) -> ()
                        n533 = local write "LPF_Filter"(w940) -> ()
                      }
                      frame #2 {
                        n534 = global read "Global_SNK3_HF.vi" "paramUnicorn"() -> (w942:T9)
                        n535 = Unbundle By Name(w942) -> ("conParam.TCP_conn"=w941:bool)
                        n536 = case shown="True" w941 {
                          frame False {
                          }
                          frame True {
                            n537 = One Button Dialog(message="Подключение к ЭБ ВЧ установлено.") -> ()  [unwired: 1 in, 1 out]
                          }
                        }
                      }
                      frame #3 {
                        n538 = control-ref of="Table"() -> (w944:refnum<vi>)
                        n539 = call "String_Indicator (SubVI).vi"("String in"=w944) -> ()  [unwired: 11 in]
                      }
                    }
                    n540 = global read "Global_SNK3_HF.vi" "GUI_AllControl"() -> (w910:refnum<vi>[])
                    n541 = call "FP_CtrlEnable (SubVI).vi"("error in"=w905, "Disabled"=T19."Enabled", "Array"=w910) -> ("error out"=w907:errorcluster)  [unwired: 8 in]
                    n542 = control-ref of="AScanXY"() -> (w909:refnum<vi>)
                    n543 = Build Array(w909) -> (w908:refnum<vi>[])
                    n544 = call "GraphLegend (SubVI).vi"("error in (no error)"=w907, "Graph"=w908) -> ("error out"=w903:errorcluster)  [unwired: 9 in]
                    n545 = Merge Errors(w904, w903) -> (w902:errorcluster)
                  }
                }
              }
              frame True {
              }
            }
            n546 = local write "Connect"(w892) -> ()
          }
          frame "Core uptime" {
            n547 = global read "Global_SNK3_HF.vi" "paramUnicorn"() -> (w950:T9)
            n548 = Unbundle By Name(w950) -> ("conParam.TCP_conn"=w949:bool)
            n549 = case shown="True" w949 {
              tunnel: [w951 w952] -> w948
              tunnel: w947 -> [w951 _]
              frame False {
              }
              frame True {
                n550 = for {
                  N: 3 -> [_]
                  tunnel: [w968] -> w953
                  stop <- w969 stop-if-true
                  n551 = global read "Global_SNK3_HF.vi" "paramUnicorn"() -> (w967:T9)
                  n552 = call "0xE3_Read_one_parameter_of_telemetry_data.vi"("Номер параметра"=1, "ParamIn"=w967) -> ("error out"=w965:errorcluster, "float number"=→"UpTime":sgl)  [unwired: 6 in, 2 out]
                  n553 = Unbundle By Name(w965) -> ("status"=w968:bool)
                  "Ошибка" <- w968
                  n554 = case shown="False" w968 {
                    frame False {
                    }
                    frame True {
                      n555 = Wait (ms)(milliseconds to wait=u32 100) -> ()  [unwired: 1 out]
                    }
                  }
                  n556 = Not(x=w968) -> (.not. x?=w969:bool)
                }
                n557 = case shown="True" w953 {
                  tunnel: [errorcluster {"status"=FALSE, "code"=0, "source"=""} ("error out") w956] -> w952
                  frame False {
                  }
                  frame True {
                    w960 = FALSE ("TCP_conn")
                    w961 = "Ошибка соединения." ("message")
                    n558 = control-ref of="Log"() -> (w962:refnum<vi>)
                    n559 = global read "Global_SNK3_HF.vi" "GUI_AllControl"() -> (w959:refnum<vi>[])
                    n560 = One Button Dialog(message=w961) -> ()  [unwired: 1 in, 1 out]
                    n561 = call "LogAdd (SubVI).vi"("string"=w961, "Log"=w962) -> ("error out"=w963:errorcluster)  [unwired: 9 in]
                    n562 = call "Disconnect (SubVI).vi"("error in"=w963, "String in"=w962) -> ("error out"=w957:errorcluster)  [unwired: 9 in]
                    n563 = call "FP_CtrlEnable (SubVI).vi"("error in"=w957, "Disabled"=T19."Disabled and Grayed Out", "Array"=w959) -> ("error out"=w956:errorcluster)  [unwired: 8 in]
                    n564 = local write "UNDT_Start"(w960) -> ()
                    n565 = local write "Connect"(w960) -> ()
                  }
                }
              }
            }
          }
          frame "ScaleOrdinate" {
            n566 = local read "ScaleOrdinate"() -> (w983:T4)
            n567 = case shown="\"дБмкВ (отн. 1 мкВ)\"" w983 {
              tunnel: ["Включено отображение данных в единицах \"отсчетах АЦП\"" ("string") "Включено отображение данных проценты полной шкалы АЦП [%]" ("string") "Включено отображение данныхв \"Вольтах\"" ("string") "Включено отображение данныхв \"дБмкВ\"" ("string")] -> w980
              tunnel: ["Отсчет АЦП [отсчет]" ("Y Scale.Name Label.Text") "Проценты полной шкалы АЦП [%]" ("Y Scale.Name Label.Text") "U [Вольт]" ("Y Scale.Name Label.Text") "дБмкВ (отн. 1 мкВ)" ("Y Scale.Name Label.Text")] -> w973
              tunnel: ["%.0f" ("Y Scale.Format String") "%.2f" ("Y Scale.Format String") "%_3p" ("Y Scale.Format String") "%_4p" ("Y Scale.Format String")] -> w972
              frame "Отсчеты АЦП (±32767)", Default {
              }
              frame "Проценты" {
              }
              frame "Вольты" {
              }
              frame "дБмкВ (отн. 1 мкВ)" {
              }
            }
            n568 = case shown="False" FALSE {
              tunnel: [0.0 w985] -> w982
              frame False {
              }
              frame True {
                n569 = local read "Gain1"() -> (w987:dbl)
                n570 = local read "Gain0"() -> (w986:dbl)
                n571 = Max & Min(x=w987, y=w986) -> (max(x,y)=w985:dbl)  [unwired: 1 out]
              }
            }
            n572 = local read "ScaleOrdinate"() -> (w978:T4)
            n573 = local read "Type_signal"() -> (w979:T7)
            n574 = call "AutoScale.vi"("ScaleOrdinate 2"=w978, "Type_signal"=w979, "UNDT_Gain"=w982) -> ("Minor"=w974:dbl, "Min"=w975:dbl, "Max"=w976:dbl)  [unwired: 6 in]
            n575 = control-ref of="Log"() -> (w981:refnum<vi>)
            n576 = call "LogAdd (SubVI).vi"("string"=w980, "Log"=w981) -> ("error out"=w971:errorcluster)  [unwired: 9 in]
            n577 = property on="AScanXY" class="XYGraph (strict)"("YScale.MinorInc"=w974, "YScale.Maximum"=w976, "YScale.Minimum"=w975, "YScale.NameLbl.Text"=w973, "YScale.FormatString"=w972) -> ()  [unwired: 2 in, 2 out]
          }
          frame "Disconnect" {
            n578 = control-ref of="Log"() -> (w1006:refnum<vi>)
            n579 = call "01_UNDT_CCEnable (SubVI).vi"("error in"=w1001, "Log"=w1006, "UNDT_Start"=FALSE ("Boolean")) -> ("error out"=w1007:errorcluster)  [unwired: 7 in, 1 out]
            n580 = call "Disconnect (SubVI).vi"("error in"=w1007, "String in"=w1006) -> ("error out"=w1002:errorcluster)  [unwired: 9 in]
            n581 = global read "Global_SNK3_HF.vi" "GUI_AllControl"() -> (w1004:refnum<vi>[])
            n582 = local write "Connect"(FALSE ("Connect")) -> ()
            n583 = call "FP_CtrlEnable (SubVI).vi"("error in"=w1002, "Disabled"=T19."Disabled and Grayed Out", "Array"=w1004) -> ("error out"=w1000:errorcluster)  [unwired: 8 in]
          }
          frame "False", Default {
          }
          frame "GIV1" {
            n584 = control-ref of="Log"() -> (w1012:refnum<vi>)
            n585 = call "06_UNDT_Pulser1Level (SubVI).vi"("error in"=w1011, "Log"=w1012, "UNDT_GIV1"="UNDT_GIV1") -> ("error out"=w1010:errorcluster)  [unwired: 8 in]
          }
          frame "GIV2" {
            n586 = control-ref of="Log"() -> (w1016:refnum<vi>)
            n587 = call "07_UNDT_Pulser2Level (SubVI).vi"("error in"=w1015, "Log"=w1016, "UNDT_GIV2"="UNDT_GIV2") -> ("error out"=w1014:errorcluster)  [unwired: 8 in]
          }
          frame "GainOffsetSlope" {
          }
          frame "HPF" {
            n588 = control-ref of="Log"() -> (w1021:refnum<vi>)
            n589 = call "04_UNDT_HPFilter (SubVI).vi"("error in"=w1020, "UNDT_HF_Filter"="UNDT_HF_Filter", "String in"=w1021) -> ("error out"=w1019:errorcluster)  [unwired: 8 in]
          }
          frame "UNDT_Freq" {
            n590 = local read "UNDT_Freq"() -> (w1025:i32)
            n591 = control-ref of="Log"() -> (w1026:refnum<vi>)
            n592 = call "24_UNDT_Freq (SubVI).vi"("error in"=w1024, "UNDT_Freq"=w1025, "String in"=w1026) -> ("error out"=w1023:errorcluster)  [unwired: 8 in]
          }
          frame "LPF" {
            n593 = control-ref of="Log"() -> (w1029:refnum<vi>)
            n594 = call "03_UNDT_LPFilter (SubVI).vi"("error in"=w1028, "LPF_Filter"="LPF_Filter", "String in"=w1029) -> ("error out"=w1027:errorcluster)  [unwired: 8 in]
          }
          frame "LoadTbl0" {
            n595 = control-ref of="Log"() -> (w1033:refnum<vi>)
            n596 = call "LoadTbl0 (SubVI).vi"("error in"=w1032, "Log"=w1033) -> ("error out"=w1031:errorcluster)  [unwired: 9 in]
          }
          frame "LoadTbl1" {
            n597 = control-ref of="Log"() -> (w1036:refnum<vi>)
            n598 = call "LoadTbl1 (SubVI).vi"("error in"=w1035, "Log"=w1036) -> ("error out"=w1034:errorcluster)  [unwired: 9 in]
          }
          frame "NTick" {
            n599 = control-ref of="Log"() -> (w1040:refnum<vi>)
            n600 = call "02_UNDT_CCTicksCount (SubVI).vi"("error in"=w1038, "UNDT_NTick"="UNDT_NTick", "String in"=w1040) -> ("error out"=w1037:errorcluster)  [unwired: 8 in]
          }
          frame "SaveParam" {
            n601 = control-ref of="Log"() -> (w1043:refnum<vi>)
            n602 = call "22_UNDT_IPSaveParam (SubVI).vi"("error in"=w1042, "String in"=w1043) -> ("error out"=w1041:errorcluster)  [unwired: 8 in, 1 out]
          }
          frame "Start" {
            n603 = control-ref of="Log"() -> (w1047:refnum<vi>)
            n604 = call "01_UNDT_CCEnable (SubVI).vi"("error in"=w1045, "Log"=w1047, "UNDT_Start"="UNDT_Start") -> ("error out"=w1044:errorcluster)  [unwired: 7 in, 1 out]
          }
          frame "Stop" {
            n605 = control-ref of="Log"() -> (w1051:refnum<vi>)
            n606 = call "01_UNDT_CCEnable (SubVI).vi"("error in"=w1049, "Log"=w1051, "UNDT_Start"=FALSE) -> ("error out"=w1048:errorcluster)  [unwired: 7 in, 1 out]
          }
          frame "Telem" {
            n607 = global read "Global_SNK3_HF.vi" "paramUnicorn"() -> (w1055:T9)
            n608 = call "0xE6_Read_all_telemetry_data.vi"("error in"=w1053, "paramUnicorn"=w1055) -> ("error out"=w1052:errorcluster, "TblTelemetry"=w1056:string[][])  [unwired: 5 in, 2 out]
            n609 = Transpose 2D Array(2D array=w1056) -> (transposed array=w1054:string[][])
            n610 = global write "Global_SNK3_HF.vi" "TblTelem"(w1054) -> ()
          }
          frame "TickInd" {
            n611 = flat-sequence {
              tunnel: w1060 -> [w1061]
              tunnel: [w1061] -> w1059
              tunnel: w1059 -> [w1064]
              tunnel: [w1063] -> w1057
              tunnel: [w1066] -> w1058
              tunnel: w1057 -> [w1066]
              frame #0 {
                n612 = local write "Ind"(FALSE ("Ind")) -> ()
              }
              frame #1 {
                n613 = call "TickInd (SubVI).vi"("error in (no error)"=w1064, "Tick"="Tick") -> ("error out"=w1063:errorcluster)  [unwired: 9 in]
              }
              frame #2 {
                n614 = local write "Ind"(TRUE ("Ind")) -> ()
              }
            }
          }
          frame "WrtTable0" {
            n615 = flat-sequence {
              tunnel: w1071 -> [w1072]
              tunnel: [w1072] -> w1070
              tunnel: w1070 -> [w1075]
              tunnel: [w1074] -> w1068
              tunnel: [w1077] -> w1069
              tunnel: w1068 -> [w1077]
              frame #0 {
                n616 = local write "Ind"(FALSE ("Ind")) -> ()
              }
              frame #1 {
                n617 = control-ref of="Log"() -> (w1076:refnum<vi>)
                n618 = call "WrtTable0 (SubVI).vi"("error in"=w1075, "Log"=w1076) -> ("error out"=w1074:errorcluster)  [unwired: 9 in]
              }
              frame #2 {
                n619 = local write "Ind"(TRUE ("Ind")) -> ()
              }
            }
          }
          frame "WrtTable1" {
            n620 = flat-sequence {
              tunnel: w1082 -> [w1083]
              tunnel: [w1083] -> w1081
              tunnel: w1081 -> [w1086]
              tunnel: [w1085] -> w1079
              tunnel: [w1088] -> w1080
              tunnel: w1079 -> [w1088]
              frame #0 {
                n621 = local write "Ind"(FALSE ("Ind")) -> ()
              }
              frame #1 {
                n622 = control-ref of="Log"() -> (w1087:refnum<vi>)
                n623 = call "WrtTable1 (SubVI).vi"("error in"=w1086, "Log"=w1087) -> ("error out"=w1085:errorcluster)  [unwired: 9 in]
              }
              frame #2 {
                n624 = local write "Ind"(TRUE ("Ind")) -> ()
              }
            }
          }
          frame "Refresh_AScan" {
            n625 = flat-sequence {
              tunnel: [w1094] -> w1093
              tunnel: w1092 -> [w1094]
              tunnel: w1093 -> [w1097]
              tunnel: [w1096] -> w1090
              tunnel: [w1099] -> w1091
              tunnel: w1090 -> [w1099]
              frame #0 {
                n626 = local write "Ind"(FALSE ("Ind")) -> ()
              }
              frame #1 {
                n627 = control-ref of="AScanXY"() -> (w1098:refnum<vi>)
                n628 = call "Refresh_AScan (SubVI).vi"("error in"=w1097, "WaveformGraph in"=w1098) -> ("error out"=w1096:errorcluster)  [unwired: 9 in]
              }
              frame #2 {
                n629 = local write "Ind"(TRUE ("Ind")) -> ()
              }
            }
          }
        }
        n630 = call <vilib>:"Simple Error Handler.vi"("type of dialog (OK msg:1)"=w851, "error in (no error)"=w852) -> ()  [unwired: 3 in, 5 out]
      }
      frame Error {
      }
    }
    n631 = global write "Global_SNK3_HF.vi" "elementGUI"(w846) -> ()
  }
  n632 = while {
    tunnel: w10 -> [w1134]
    tunnel: w7 -> [w1133]
    tunnel: [w1132] -> w9
    stop <- w1107 stop-if-true
    w1110 = T31 {"UNDT_Type_signal"=enum."РЧ сигнал", "ФНЧ"=TRUE, "UNDT_Mean"=1, "IIR filter"={"Topology"=enum."Butterworth", "Type"=enum."Bandpass", "Order"=4, "Lower Fc"=200000.0, "Upper Fc"=10000000.0, "PB Ripple"=1.0, "SB Attenuation"=60.0}, "ZeroDimension"=4000, "ТипДетектора"=enum."Оконный детектор", "FilterCor"={"HPFFilterNum"=enum."HPF_OFF", "LPFBode"=[], "HPFBode"=[], "EnableFilterСorrect"=TRUE, "LPF_Filter"=enum."14 МГц"}, "MeasControl"={"approx freq"=0.0, "search (+/- % of Fsampl.)"=1.0, "start, duration"={"start samples/time"=-1.0, "duration"=0.0, "EnableSubset"=TRUE}, "averaging type"=enum."Linear", "window"=enum."Rectangular (none)", "hysteresis"=0.0, "level"=0.0}}  # Parameters
    n633 = Dequeue Element(queue=w1134, error in (no error)=w1133) -> (element=w1106:T16, error out=w1132:errorcluster)  [unwired: 3 out]
    n634 = Not(x="Pause") -> (.not. x?=w1103:bool)
    n635 = global read "Global_SNK3_HF.vi" "Ind"() -> (w1102:bool)
    n636 = And(x=w1103, y=w1102) -> (x .and. y?=w1105:bool)
    n637 = local read "HPF_Bode"() -> (w1122:cluster{"Frq":dbl[], "Kt":dbl[]}[])
    n638 = local read "LPF_Bode"() -> (w1121:cluster{"Frq":dbl[], "Kt":dbl[]}[])
    n639 = local read "LPF_Filter"() -> (w1120:enum16{"14 МГц", "10 МГц", "7.5 МГц"})
    n640 = local read "UNDT_HF_Filter"() -> (w1119:u16)
    n641 = expression code="x*1e6"("FreqFind") -> (w1115:dbl)
    n642 = case shown="\"Выкл.\"" "HPF_Filter_Prog" {
      tunnel: [400000.0 ("Lower Fc") 100000.0 ("Lower Fc") 800000.0 ("Lower Fc") 1500000.0 ("Lower Fc") 2000000.0 ("Lower Fc")] -> w1130
      frame "0.4 МГц", Default {
      }
      frame "Выкл." {
      }
      frame "0.8 МГц" {
      }
      frame "1.5 МГц" {
      }
      frame "2.0 МГц" {
      }
    }
    n643 = Bundle By Name(cluster=T30 {"approx freq"=-1.0, "search (+/- % of Fsampl.)"=0.1, "start, duration"={"start samples/time"=0.0, "duration"=1.0, "EnableSubset"=FALSE}, "averaging type"=enum."Linear", "window"=enum."Rectangular (none)", "hysteresis"=0.0, "level"=0.0} ("MeasControl"), "approx freq"=w1115, "start, duration"="StartLen", "level"="TrigLevel") -> (w1116:T30)
    n644 = Bundle By Name(cluster=T29 {"HPFFilterNum"=enum."HPF_OFF", "LPFBode"=[], "HPFBode"=[], "EnableFilterСorrect"=TRUE, "LPF_Filter"=enum."14 МГц"} ("FilterCor"), "HPFBode"=w1122, "LPFBode"=w1121, "LPF_Filter"=w1120, "HPFFilterNum"=w1119, "EnableFilterСorrect"="FiltrCor") -> (w1131:T29)
    n645 = Bundle By Name(cluster="IIR filter", "Lower Fc"=w1130) -> (w1117:T8)
    n646 = Bundle By Name(cluster=w1110, "UNDT_Type_signal"="Type_signal", "ФНЧ"="Видеофильтр", "UNDT_Mean"="UNDT_Mean", "IIR filter"=w1117, "ZeroDimension"="ZeroDimensionDetect", "ТипДетектора"="Тип детектора", "FilterCor"=w1131, "MeasControl"=w1116) -> (w1108:T31)
    n647 = case shown="True" w1105 {
      tunnel: w1106 -> [_ w1157]
      tunnel: w1108 -> [_ w1156]
      frame False {
      }
      frame True {
        n648 = Unbundle By Name(w1157) -> ("UNDT_Cluster.N tick"=w1135:u8, "UNDT_Cluster"=w1137:T17)
        n649 = call "Graph (SubVI).vi"("MeasChanel"=u32[] [0, 1], "Parameters"=w1156, "DataIn"=w1157) -> ("Meas"=w1152:T32, "Filtered X"=w1143:dbl[])  [unwired: 7 in]
        n650 = local read "UNDT_meas"() -> (w1150:string[][])
        n651 = Unbundle By Name(w1137) -> ("Overload"=w1136:bool)
        n652 = call "t0 dt (SubVI).vi"("ScaleAbciss"="ScaleAbciss", "speed"="speed", "UNDT_Cluster"=w1137) -> ("magnitude"=w1155:cluster{"t0":dbl, "dt":dbl, "magnitude":dbl[]})  [unwired: 8 in]
        n653 = Bundle By Name(cluster=w1155, "magnitude"=w1143) -> (w1148:cluster{"t0":dbl, "dt":dbl, "magnitude":dbl[]})
        n654 = call "MeasToTable (SubVI).vi"("UNDT_NTick"=1, "Meas"=w1152, "N tick"=w1135, "Table"=w1150) -> ("TableOut"=w1140:string[][])  [unwired: 7 in]
        "UNDT_meas" <- w1140
        n655 = global write "Global_SNK3_HF.vi" "UNDT_meas"(w1140) -> ()
        n656 = global read "Global_SNK3_HF.vi" "AScanOscNum"() -> (w1141:u8)
        n657 = local read "Overload"() -> (w1139:bool[])
        n658 = local read "AScanXY"() -> (w1146:T1)
        n659 = call "InterpolationAScan (SubVI).vi"("Interpolation factor (n)"="Interpolation factor (n)", "magnitude"=w1148) -> ("XY Graph"=w1144:cluster{dbl[], dbl[]})  [unwired: 9 in]
        n660 = Equal?(x=w1135, y=w1141) -> (x = y?=w1142:bool)
        n661 = case shown="False" w1142 {
          tunnel: w1143 -> [w1159 _]
          frame True {
            n662 = global write "Global_SNK3_HF.vi" "AScanOsc"(w1159) -> ()
          }
          frame False {
          }
        }
        n663 = in-place {
          in-place-border: w1136 -> [w1158]
          n664 = in-place-array #1(w1139, w1135) -> ()  [unwired: 1 out]
          n665 = in-place-array #1(w1158) -> (w1138:bool[])  [unwired: 1 out]
        }
        n666 = in-place {
          in-place-border: w1144 -> [w1160]
          n667 = in-place-array #2(w1146, w1135) -> ()  [unwired: 1 out]
          n668 = in-place-array #2(w1160) -> (w1145:T1)  [unwired: 1 out]
        }
        n669 = local write "Overload"(w1138) -> ()
        n670 = local write "AScanXY"(w1145) -> ()
      }
    }
    n671 = global read "Global_SNK3_HF.vi" "Stop"() -> (w1107:bool)
  }
  n672 = call "Queue_Status (SubVI).vi"("error in (no error)"=w7, "Queue in"=w10) -> ("error out"=w11:errorcluster)  [unwired: 9 in]
  n673 = call "UDP1in (SubVI).vi"("error in (no error)"=w7, "Queue in"=w10) -> ("error out"=w15:errorcluster)  [unwired: 9 in]
  n674 = call "UDP2in (SubVI).vi"("error in (no error)"=w7, "Queue in"=w10) -> ("error out"=w14:errorcluster)  [unwired: 9 in]
  n675 = Release Queue(queue=w5, error in (no error)=w17) -> (error out=w8:errorcluster)  [unwired: 1 in, 2 out]
  n676 = Merge Errors(w11, w15, w14, w9, w8) -> (w16:errorcluster)
  n677 = call <vilib>:"Simple Error Handler.vi"("type of dialog (OK msg:1)"=w19, "error in (no error)"=w16) -> ()  [unwired: 8 out]
